vi "AlliGator GUI Actions.vi"(0 "AlliGator Q Elements in":T6[](array[typedef]), 1 "VI in":refnum<vi>, 2 "Script":bool, 5 "AlliGator IV DVR":refnum<data-value>, 7 "AlliGator Q Event in":T7=enum."GUI:Idle", 9 "Data":variant, 11 "error in (no error)":errorcluster, 12 "AlliGator Ctrl Refnums":T8) -> (3 "Script?":bool, 4 "AlliGator Q Elements out":T6[](array[typedef]), 6 "AlliGator IV DVR":refnum<data-value>, 10 "[Notebook Message]":T1[](array[typedef]) {"Message Style"."Font Size" min=6.0 step=1.0}, 14 "Quit?":bool, 15 "error out":errorcluster)   [LabVIEW 2021, in "AlliGator Action Engine.lvlib"]
doc: "Processes AlliGator GUI-related actions."
uses:
  AlliGator Action Engine.lvlib
  Internal Variables/AlliGator Internal Variables v2.ctl
  <vilib>/vision/Image Controls.llb/IMAQ Image.ctl
  Internal Variables/AlliGator Gate Image Set.ctl
  Files/AlliGator FLI Dataset Type.ctl
  Files/AlliGator Data Series Type.ctl
  Dual-Channel Datasets/AlliGator Dataset Channel.ctl
  Settings/AlliGator Gate Arithmetic.ctl
  Source Image/AlliGator Displayed Image.ctl
  Image/Named ROI Description.ctl
  Phasor Graph/AlliGator Decay Metadata v3.ctl
  Decay Analysis/Decay Preprocessing/AlliGator Decay Background Subtraction Info.ctl
  Decay Analysis/Decay Preprocessing/AlliGator Baseline Subtraction Method.ctl
  Graphs/XY Graph/XY Graph Plot Shift Parameters.ctl
  Graphs/XY Graph/XY Graph Plot Shift Method.ctl
  Decay Analysis/Decay Preprocessing/AlliGator Decay Extrapolation Parameters.ctl
  Phasor/Calibration Phasor (m, phi).ctl
  Phasor/Phasor Reference Series.ctl
  Phasor/Phasor Calibration Map v2.ctl
  Phasor/Phasor (g, s).ctl
  Phasor Graph/AlliGator Raw Phasor Plot Data v5.ctl
  Phasor/Phasor Standard Deviation Options.ctl
  Phasor Plot/AlliGator Phasor Multi-Harmonic Data.ctl
  Phasor/Phasor Harmonic Data.ctl
  Decay Fit Parameter Map/AlliGator Decay Fit Options & Parameters v4.ctl
  Fits/IRF(X)PSED/Decay Fit Options v4.ctl
  Fits/Decay Convolution/Decay Model.ctl
  Fits/Residual Type.ctl
  Fits/IRF(X)PSED/Fit Weights Type v2.ctl
  Fits/Non-linear Fitting Method v2.ctl
  Fits/Fit Calculation Method.ctl
  Fits/Non-linear Fitting Algorithm.ctl
  Decay Analysis/Decay Fit/AlliGator Decay Fit Parameter Constraints 2.ctl
  Fits/IRF(X)PSED/Decay Fit Parameters In List.ctl
  Fits/IRF(X)PSED/MLE Baseline Offset Type.ctl
  Decay Analysis/Decay Preprocessing/AlliGator Decay Preprocessing Parameters.ctl
  Fits/IRF(X)PSED/Decay Fit Parameters & Derived Quantities List v2.ctl
  Fits/IRF(X)PSED/Decay Fit Result Constraint.ctl
  Decay Fit Parameter Map/AlliGator Parameter Maps Data.ctl
  AlliGator Q Event.ctl
  GUI/AlliGator Ctrl Refnums.ctl
  GUI/AlliGator Other Ctrl Refnums.ctl
  GUI/AlliGator State Indicator.ctl
  GUI/AlliGator Main Window Tabs.ctl
  GUI/AlliGator Phasor Plot Ctrl Refnums.ctl
  GUI/AlliGator Phasor Graph Ctrl Refnums.ctl
  Phasor/Phasor Calibration Type.ctl
  GUI/AlliGator Dataset Ctrl Refnums.ctl
  GUI/AlliGator Registered Events Ctrl Refnums.ctl
  GUI/AlliGator Image Histogram Control Refnums.ctl
  Histograms/Linear Histogram Options.ctl
  Histograms/Histogram Bin Option.ctl
  Histograms/Histogram Bin Position.ctl
  Decay Fit Parameter Map/AlliGator Decay Fit Map Control Refnums.ctl
  Parameter Map/AlliGator Parameter Map Control Refnums.ctl
  AlliGator Q Element.ctl
  Notebook/Notebook Message Object.ctl
  Rich Text Box/Text Formatting.ctl
  Rich Text Box/Text Colors.ctl
  Rich Text Box/Text Style.ctl
  Rich Text Box/Text Alignment.ctl
  Rich Text Box/Text Format List.ctl
  Globals, Variables, Constants/AlliGator Variables List.ctl
  Settings/AlliGator Settings List.ctl
  Alligator Elements Order in Action Stack.ctl
  GUI/AlliGator Open Wndow Event Data.ctl
  GUI/AlliGator Windows List.ctl
  GUI/Open VI Options.ctl
  GUI/Embedded Progress Bar Q Element.ctl
  AlliGator State Indicators List.ctl
  GUI/AlliGator Set State Indicator Data.ctl
  Test Suites/AlliGator Test Data.ctl
  Globals, Variables, Constants/AlliGator Globals.vi
  Globals, Variables, Constants/AlliGator Abort.vi
  Variant/Variant to Data/Variant to Boolean.vi
  Fits/Abort Fit Global.vi
  Variant/Variant to Data/Variant to U16.vi
  Variant/Variant to Data/Variant to String.vi
  Variant/Variant to Data/Variant to I32.vi
  Source Image/AlliGator Source Image.lvlib
  GUI/AlliGator GUI.lvlib
  Globals, Variables, Constants/AlliGator Globals, Variables & Constants.lvlib
  Variant/Variant to Data/Variant to Data.lvlib
  Internal Variables/AlliGator Internal Variables.lvlib
  GUI/GUI.lvlib
  ROIs/AlliGator ROIs.lvlib
  Strings/Strings.lvlib
  Settings/AlliGator Settings.lvlib
  Notebook/Notebook.lvlib
  Scripts/AlliGator Scripts.lvlib
  Python Plugins API/AlliGator Python Plugins.lvlib
  Fits/Fits.lvlib
  Utilities/Utilities.lvlib
  Sound/Sound.lvlib
  Formula/Formula.lvlib
  Test Suites/AlliGator Test Suite.lvlib
  Phasor/Phasor.lvlib
  Image/Image.lvlib
  Decay Analysis/Decay Preprocessing/AlliGator Decay Preprocessing.lvlib
  Graphs/XY Graph/XY Graph Add-Ons.lvlib
  Phasor Graph/AlliGator Phasor Graph.lvlib
  Files/AlliGator Files.lvlib
  Phasor Plot/AlliGator Phasor Plot.lvlib
  Decay Analysis/Decay Fit/AlliGator Decay Fit.lvlib
  Decay Fit Parameter Map/AlliGator Decay Fit Parameter Map.lvlib
  Rich Text Box/Rich Text Box.lvlib
  Dual-Channel Datasets/AlliGator Dual-Channel Datasets.lvlib
  Histograms/Histogram Window.lvlib
  Parameter Map/AlliGator Parameter Map.lvlib
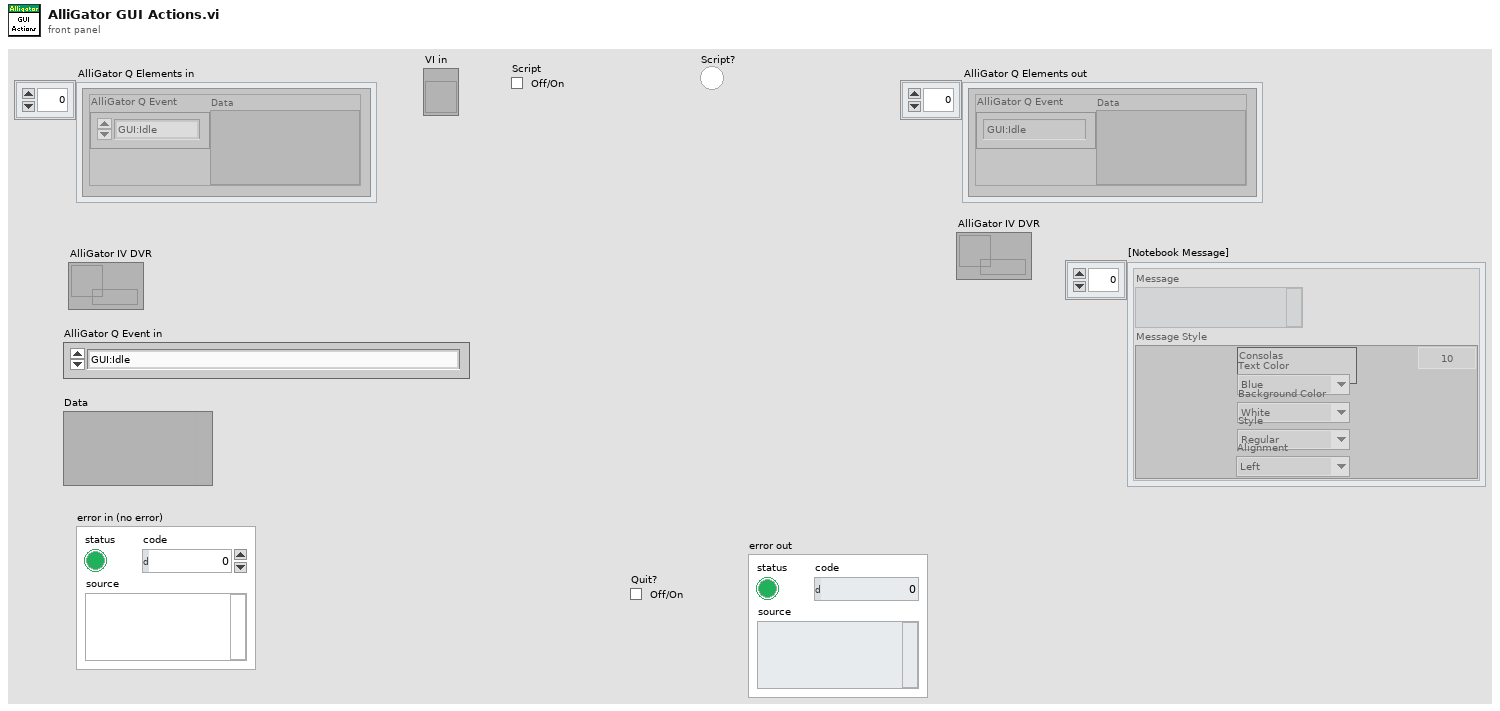
[diagram p1: front panel]
types:
  T1 = typedef "Notebook.lvlib/Notebook Message Object.ctl" = cluster{"Message":string, "Message Style":T2}
  T2 = typedef "Rich Text Box.lvlib/Text Formatting.ctl" = cluster{"Font":string, "Text Color":T3, "Background Color":T3, "Style":T4, "Font Size":dbl, "Alignment":T5}
  T3 = typedef "Rich Text Box.lvlib/Text Colors.ctl" = enum16{"Unchanged", "Black", "Blue", "Cyan", "Maroon", "Gray", "Violet", "Green", "Light Green", "Orange", "Yellow", "Magenta", "Red", "White"}
  T4 = typedef "Rich Text Box.lvlib/Text Style.ctl" = enum16{"Regular", "Bold", "Italic", "Underline", "Strikeout"}
  T5 = typedef "Rich Text Box.lvlib/Text Alignment.ctl" = enum16{"Left", "Right", "Center"}
  T6 = typedef "AlliGator Action Engine.lvlib/AlliGator Q Element.ctl" = cluster{"AlliGator Q Event":T7, "Data":variant}
  T7 = typedef "AlliGator Action Engine.lvlib/AlliGator Q Event.ctl" = enum16{"---- Files ----", "Files:Set Batch Export Files To Save", "Files:Set Dataset Loading & Pre-processing Options", "Files:Check #Frames in Dataset", "Files:Increment Frame Index", "Files:Open Mask Image", "Files:Open White Light Image", "Files:Open Single Dataset", "Files:New Folder of Folders Selected", "Files:Load File (all Types)_Scriptable", "Files:Move Flattened Series to Folders Series", "Files:Select Folder", "Files:Load FLI Dataset", "Files:Load Swiss SPAD 1 Dataset", "Files:Load Swiss SPAD 2 Dataset", "Files:Load .sdt FLI Dataset", "Files:Load .ptu FLI Dataset", "Files:Load .bin FLI Dataset", "Files:Load Single Gate Image Folder", "Files:Load I/m/phi Dataset (deprecated)", "Files:Load Single Image", "Files:Subtract Background File", "Files:Export FLI Dataset", "Files:Load HDF5 FLI Dataset", "Files:Set Destination File Path", "Files:Save Mask Image", "Files:Batch Conversion", "Files:New Folder Selected", "Files:Close FLI Dataset", "Files:Close FLI Dataset Series", "Files:Close White Light Image", "Files:Close Mask Image", "---- FLI Dataset ----", "FLI Dataset:Channel Arithmetic", "FLI Dataset:Export Average Lifetime Map as ASCII", "FLI Dataset:Export User-Defined Quantity Map as ASCII", "FLI Dataset:Python Function FLI Dataset Event", "FLI Dataset:ROI Analysis", "FLI Dataset:Tilted Logistic Square Gated IRF Characteristics Map", "FLI Dataset:Logistic Square Gated IRF Characteristics Map", "FLI Dataset:Square Gated IRF Characteristics Map", "FLI Dataset:Multi-ROI Single-Pixel Phasor Analysis", "FLI Dataset:Multi-ROI Single-Pixel NLSF Analysis", "FLI Dataset:All ROIs IRF Extraction", "FLI Dataset:All ROIs Decay Fit Non-Interactive (Fast + Individual IRF)", "FLI Dataset:All ROIs Phasor Analysis", "FLI Dataset:All ROIs Decay Fit", "FLI Dataset:Fluorescence Decay Statistics", "FLI Dataset:Update Decay Statistics Graph", "FLI Dataset:Get Decay from ROI", "FLI Dataset:All ROIs Average Lifetimes", "FLI Dataset:Save/Load Local IRFs", "FLI Dataset:Clear Local IRFs", "FLI Dataset:Phasor Calibration Maps (# Gates Series) Script", "FLI Dataset:Calibrated Phasor Map Series", "---- FLI Dataset Series ----", "FLI Dataset Series:Sum All Datasets in Series", "FLI Dataset Series:Add Dataset to Accumulated Dataset", "FLI Dataset Series:Display Accumulated Dataset", "FLI Dataset Series:Clear Dataset Series Sum", "FLI Dataset Series:Time-Series Analysis (NLSF)", "FLI Dataset Series:Time-Series Analysis (Phasor)", "---- Image ----", "Image:Update Image Profile Plots", "Image:Image Histogram Cursor Move", "Image:Image Histogram", "Image:Image Contrast", "Image:Set Image Histogram Cursor Move Flag", "Image:Clear Image Overlay", "Image:Use ROI as Search Area", "Image:Set ROI Diameter", "Image:Save Image Data as TIFF", "Image:Save Displayed Image with Overlay", "Image:Save Image Overlay Only", "Image:Save Image as Hot Pixel Mask", "Image:Change Source Image Color Palette", "Image:Copy Image to Clipboard", "Image:Source Image ROI Selection", "Image:Delete All ROIs", "Image:Delete All Unselected ROIs", "Image:Delete ROI", "Image:Merge All ROIs", "Image:Store ROI", "Image:Source Image ROI Storage", "Image:Export ROI Description to Notebook", "Image:Save ROI", "Image:Load ROI", "Image:Paste ROI Definition", "Image:Clear ROI", "Image:Identify ROIs in Mask Image", "Image:Create Complementary ROI", "Image:Create Contour ROI", "Image:Create ROI(s) from Pixels with Peak above Min_Scriptable", "Image:Create ROI(s) from Pixels with Intensity above Min_Scriptable", "Image:Compute ROI Statistics", "Image:Delete ROI(s) based on ROI Characteristics", "Image:Create ROI Grid", "Image:ROI to Individual Pixel ROIs", "Image:Python Function Source Image Event", "Image:Show Phasor Calibration Map ROI Centers", "Image:Convert ROI to Mask Image", "Image:Mouse Move", "Image:Mouse Up", "Image:Set Source Image Mouse Move Flag", "Image:Add Scale Bar Overlay", "Image:Delete Existing ROIs Option", "Image:Overlay ROI Median", "Image:Check Current ROI", "Image:Update True Pixel Value", "---- Decay ----", "Decay:Clear IRF/Reference Plot", "Decay:Add Decay to Graph", "Decay:Smoothen Plot", "Decay:Smoothen Plot Tail", "Decay:Average Selected Plots", "Decay:Extract IRF", "Decay:Optimal IRF Extraction", "Decay:Threshold IRF", "Decay:Fit to Model IRF", "Decay:Fit IRF to Square Gate", "Decay:Fit IRF to Logistic Square Gate", "Decay:Fit IRF to Tilted Logistic Square Gate", "Decay:Create Bounding Cursors Set", "Decay:Export Bounding Cursors Definition to Notebook", "Decay:Denoise Plot", "Decay:Compute Cumulative Function", "Decay:Use as Reference Decay", "Decay:Show Reference Decay/IRF", "Decay:Extrapolate Decay", "Decay:Create Head & Tail Bounding Cursors", "Decay:Store Cursor-defined Head & Tail Fractions", "Decay:Rebin Plot", "Decay:1-Normalize Decay", "Decay:[0-1]-Normalize Plot", "Decay:Straighten Decay", "Decay:Shift Decay", "Decay:Fold Decay", "Decay:Fit Decay", "Decay:Global Fit of Selected Decays", "Decay:Post Global Fit Script", "Decay:Add Global Fit Parameters to Graph", "Decay:Add Decay Parameter(s) to Plot (Graph)", "Decay:Export Decay to Phasor Graph", "Decay:Compute Average Lifetime", "Decay:Plot Convolution", "Decay:Graph Tip Strip Update", "---- Decay Statistics ----", "Decay Statistics:Tip Strip Update", "---- Intensity Time Trace ----", "Intensity Time Trace:Use File Timestamp", "Intensity Time Trace:Load Intensity Corrections File", "Intensity Time Trace:Clear Intensity Corrections File", "Intensity Time Trace:Tip Strip Update", "---- Phasor Plot ----", "Phasor Plot:Build Phasor Plot", "Phasor Plot:Change Phasor Plot Color Palette", "Phasor Plot:Adjust Phasor Plot Display Range", "Phasor Plot:Highlight Image ROI in Phasor Plot", "Phasor Plot:Save Phasor Plot Image with Overlay", "Phasor Plot:Export Complex Phasor Map", "Phasor Plot:Export Phasor Ratio Map", "Phasor Plot:Export Average Lifetime Map", "Phasor Plot:Compute Phase Lifetime Histogram", "Phasor Plot:Compute Phasor Ratio Histogram", "Phasor Plot:Compute Phase Lifetime vs Intensity Scatter Plot", "Phasor Plot:Weber 2-Component Decomposition", "Phasor Plot:Update Phasor Color Map Vertices", "Phasor Plot:Clear Phasor Overlay", "Phasor Plot:Use Segment Extremities as References", "Phasor Plot:Use UC/Segment Intersections as References", "Phasor Plot:Use UC/Principal Axis Intersections as References", "Phasor Plot:Use UC/Linear Fit Intersections as References", "Phasor Plot:Update Phasor Plot Reference", "Phasor Plot:Show Local Phasor Info in Phasor Plot", "Phasor Plot:Update Phasor Plot State", "Phasor Plot:Phasor Plot ROI Storage", "Phasor Plot:Phasor Plot ROI Selection", "Phasor Plot:Python Function Phasor Plot Event", "Phasor Plot:Overlay Phasor ROI, Ratio or Map in Source Image", "Phasor Plot:Compute Decay of Selected Phasors", "Phasor Plot:Phasor at Image Pixel", "Phasor Plot:Mouse Move", "Phasor Plot:Mouse Up", "Phasor Plot:Display Range Mouse Move", "Phasor Plot:Set Mouse Move Flag", "Phasor Plot:Update True Phasor Plot Value", "---- Phasor Graph ----", "Phasor Graph:Get Phasor Value", "Phasor Graph:Create New Phasor Plot Dialog", "Phasor Graph:Update Last Phasor Value", "Phasor Graph:Update Phasor (m, phi)", "Phasor Graph:Remove Single Phasor from Plot", "Phasor Graph:Add Single Phasor to Plot", "Phasor Graph:Remove Phasor Plot", "Phasor Graph:Remove Selected Phasor Plots", "Phasor Graph:Clear Phasor Data", "Phasor Graph:Clear Phasor Graph", "Phasor Graph:Cursor Move", "Phasor Graph:Draw Cursor Connecting Line", "Phasor Graph:Clear Cursor Connecting Line", "Phasor Graph:Find UC Intersection", "Phasor Graph:Use UC/Cursor-Defined Line Intersections", "Phasor Graph:Use Selected Plots Fitted Line/UC Intersections", "Phasor Graph:Use Selected Plots Principal Axis/UC Intersections", "Phasor Graph:Show Single Phasor", "Phasor Graph:Save Single Phasor Plot", "Phasor Graph:Save All Phasor Plots", "Phasor Graph:Load Phasor Plot(s)", "Phasor Graph:Phasor Multiplication", "Phasor Graph:Compute Average Phasor", "Phasor Graph:Compute Multiple Average Phasors (Selected Plots)", "Phasor Graph:Export Single Phasor Plot Phase Lifetimes", "Phasor Graph:Parameter 2 vs Parameter 1 Scatter Plot", "Phasor Graph:Use Cursor n Location", "Phasor Graph:Set Reference n to Current Phase Lifetime Value", "Phasor Graph:Set Reference n to Lifetime Value", "Phasor Graph:Set Cursor n Location", "Phasor Graph:Save Phasor Graph Image", "Phasor Graph:Update SEPL Plot", "Phasor Graph:Export Single Phasor Plot Data", "Phasor Graph:Export Selected Phasor Plots Data", "Phasor Graph:Python Function Phasor Graph Event", "Phasor Graph:Tip Strip Update", "---- Calibration ----", "Calibration:Set Calibration Type", "Calibration:Load/Save Phasor Calibration", "Calibration:Load/Save Phasor Calibration Series", "Calibration:Load/Save Phasor Calibration Map", "Calibration:Use as Calibration", "Calibration:Compute Optimal Calibration from Phasor References", "Calibration:Clear Phasor Calibration", "Calibration:Single Phasor Calibration Information", "Calibration:Use as Calibration Series", "Calibration:Use as Calibration Map", "Calibration:Clear Calibration Series", "Calibration:Phasor Calibration Series Information", "Calibration:Clear Calibration Map", "Calibration:Phasor Calibration Map Information", "Calibration:Apply Phasor Calibration", "Calibration:Update Single Plot Calibration", "Calibration:Update Multiple Plots Calibration", "Calibration:Clear Single Plot Calibration", "Calibration:Clear All Plots Calibrations", "Calibration:Clear Plot(s) Calibration(s)?", "---- Phasor Ratio ----", "Phasor Ratio:Clear Reference n", "Phasor Ratio:Toggle Selected Plot(s)  Lock to Reference 1", "Phasor Ratio:Use as Reference n", "Phasor Ratio:Send Reference n to Notebook", "Phasor Ratio:Toggle Selected Plot(s)  Lock to Reference 2", "Phasor Ratio:Compute Phasor Ratio at Mouse Location", "Phasor Ratio:Compute Phasor Plot's Average Phasor Ratio", "Phasor Ratio:Compute Time-Series Phasor Ratios", "Phasor Ratio:Fit Line to Phasor Ratio Plot", "Phasor Ratio:Save References", "Phasor Ratio:Load References", "Phasor Ratio:Update Phasor Reference 1", "Phasor Ratio:Update Phasor Reference 2", "Phasor Ratio:Move Cursor n to Reference n", "Phasor Ratio:Use as Phasor Reference 1 Lifetime", "Phasor Ratio:Use as Phasor Reference 2 Lifetime", "Phasor Ratio:Export Phasor Ratio Map as ASCII", "Phasor Ratio:Tip Strip Update", "---- Lifetime & Other Parameters Graph ----", "Lifetime:Compute Sliced Mean, SDV and CV Plots", "Lifetime:Plot Decay Shifts", "Lifetime:Plot Histogram", "---- Decay Fit Parameter Map ----", "Decay Fit Parameter Map:Export ROI NLSF Data as ASCII", "Decay Fit Parameter Map:Set Decay Fit Parameter Map Selection", "Decay Fit Parameter Map:Build Decay Fit Parameter Map", "Decay Fit Parameter Map:Change Decay Fit Parameter Map Color Palette", "Decay Fit Parameter Map:Export Decay Fit Parameter Map Data as ASCII", "Decay Fit Parameter Map:Export All Decay Fit Parameter Maps Data as ASCII", "Decay Fit Parameter Map:Selected Parameter Scatterplot", "Decay Fit Parameter Map:Parameter 2 vs Parameter 1 Scatterplot", "Decay Fit Parameter Map:Save Decay Fit Parameter Map Image", "Decay Fit Parameter Map:Save-Load IRFs & Fit Data", "Decay Fit Parameter Map:Update Local Decay Plots", "Decay Fit Parameter Map:Python Function Decay Fit Parameters Map Event", "Decay Fit Parameter Map:Overlay Decay Fit Parameter Map in Source Image", "Decay Fit Parameter Map:Selected Parameter vs Intensity Scatterplot", "Decay Fit Parameter Map:Mouse Up", "Decay Fit Parameter Map:Mouse Move", "Decay Fit Parameter Map:Display Range Mouse Move", "Decay Fit Parameter Map:Change Map Resolution", "Decay Fit Parameter Map:Variance Significance Maps", "Decay Fit Parameter Map:Fit Result Constraints Window", "---- Parameter Map ----", "Parameter Map:Export ROI Parameters Data as ASCII", "Parameter Map:Add Parameter Map Set", "Parameter Map:Delete Parameter Map Set", "Parameter Map:Update Parameter List", "Parameter Map:Build Parameter Map", "Parameter Map:Change Parameter Map Color Palette", "Parameter Map:Export Parameter Map Data as ASCII", "Parameter Map:Export All Parameter Maps Data as ASCII", "Parameter Map:Selected Parameter Scatterplot", "Parameter Map:Parameter 2 vs Parameter 1 Scatterplot", "Parameter Map:Selected Parameter vs Intensity Scatterplot", "Parameter Map:Save Parameter Map Image", "Parameter Map:Save-Load IRFs & Parameter Maps (TODO)", "Parameter Map:Set Parameter Map Selection", "Parameter Map:Python Function Parameter Map Event", "Parameter Map:Overlay Parameter Map in Source Image", "Parameter Map:Update Local Decay Plots", "Parameter Map:Mouse Up", "Parameter Map:Mouse Move", "Parameter Map:Display Range Mouse Move", "---- Generic Graph ----", "Generic Graph:Generic XY Graph Event", "Generic Graph:Python Function XY Graph Event", "Generic Graph:New Plot", "Generic Graph:Save Plot", "Generic Graph:XY Plot Histogram", "Generic Graph:Set XY Graph Plot Name", "Generic Graph:Set Last Cursor Style", "Generic Graph:Tip Strip Update", "---- GUI ----", "GUI:Start Script", "GUI:Type of Displayed Image Changed", "GUI:Gate Image Slide Changed", "GUI:Show Busy Icon", "GUI:Show Busy Icon & Abort Button", "GUI:Hide Busy Icon", "GUI:Hide Busy Icon & Abort Button", "GUI:Abort", "GUI:End Script", "GUI:Start Timing", "GUI:End Timing", "GUI:Set State Indicator", "GUI:Send Parameters JSON Strings to Clipboard", "GUI:Set Gate Step", "GUI:Idle", "GUI:Initialization", "GUI:Quit", "GUI:Increment Dataset Index", "GUI:Set Dataset Index to -1", "GUI:Time Series Slider Moved", "GUI:Time Series Slider Changed", "GUI:Toggle Playback or Loop", "GUI:Playback Script", "GUI:Set Phasor Frequency", "GUI:Open Window", "GUI:Start Test Script", "GUI:End Test Script", "GUI:Set Verbose Mode", "GUI:Set Verbose Settings Mode", "DEBUG"}
  T8 = typedef "AlliGator GUI.lvlib/AlliGator Ctrl Refnums.ctl" = cluster{"Other AlliGator Ctrl Refnums":T9, "Phasor Plot Ctrl Refnums":T10, "Phasor Graph Ctrl Refnums":T11, "Dataset Control Refnums":T12, "Registered Events Ctrl Refnums":T13, "Image Histogram Ctrl Refnums":T14, "Decay Fit Map Ctrl Refnums":T15, "Parameter Map Ctrl Refnums":T16}
  T9 = typedef "AlliGator GUI.lvlib/AlliGator Other Ctrl Refnums.ctl" = cluster{"State Indicators":refnum<vi>, " Progress Bar":refnum<vi>, "Decay Graph Active":refnum<vi>, "Decay Statistics Bin":refnum<vi>, "Time Step":refnum<vi>, "Use File Timestamp":refnum<vi>, "Tab Control":refnum<vi>, "CPU":refnum<vi>, "Abort Fit":refnum<vi>, "Dataset File/Folder Path":refnum<vi>, "Abort ROI Creation":refnum<vi>, "Event LED":refnum<vi>, "Dataset File/Folder Path 2":refnum<vi>, "Dataset File/Folder Path 3":refnum<vi>, "Dataset File/Folder Path 4":refnum<vi>, "Dataset File/Folder Path 5":refnum<vi>, "Dataset File/Folder Path 6":refnum<vi>, "Dataset File/Folder Path 7":refnum<vi>, "Dataset File/Folder Path 8":refnum<vi>, "Dataset File/Folder Path 9":refnum<vi>, "Dataset File/Folder Path 10":refnum<vi>, "Dataset File/Folder Path 11":refnum<vi>}
  T10 = typedef "AlliGator GUI.lvlib/AlliGator Phasor Plot Ctrl Refnums.ctl" = cluster{"Phasor Ratio":refnum<vi>, "Modulus Lifetime":refnum<vi>, "Phasor at cursor (m, phi)":refnum<vi>, "Phase Lifetime":refnum<vi>, "Phasor at cursor (g, s)":refnum<vi>, "Phasor Plor Average Lifetime":refnum<vi>, "Phasor Plot Active":refnum<vi>, "Save Phasor Plot":refnum<vi>, "Image Overlay Color":refnum<vi>, "Phasor Plot Color Scale":refnum<vi>, "Reference 1 Button":refnum<vi>, "Reference 2 Button":refnum<vi>, "True Phasor Plot Value":refnum<vi>}
  T11 = typedef "AlliGator GUI.lvlib/AlliGator Phasor Graph Ctrl Refnums.ctl" = cluster{"Phasor Ratio":refnum<vi>, "Modulus Lifetime":refnum<vi>, "Phasor at cursor (m, phi)":refnum<vi>, "Phase Lifetime":refnum<vi>, "Phasor at cursor (g, s)":refnum<vi>, "Phasor Graph Average Lifetime":refnum<vi>, "Phasor Graph Active":refnum<vi>, "Save Phasor Graph":refnum<vi>, "Phasor Frame Slide":refnum<vi>, "Single Step Phasor":refnum<vi>, "Calibration Type":refnum<vi>, "Show Line":refnum<vi>, "Phase Lifetime 1":refnum<vi>, "Phase Lifetime 2":refnum<vi>, "Phasor Graph Frequency":refnum<vi>, "Phasor Reference 1 Control":refnum<vi>, "Phasor Reference 2 Control":refnum<vi>, "Calibration Lifetime":refnum<vi>, "Phase Lifetime SDV":refnum<vi>, "Average Lifetime SDV":refnum<vi>, "Phasor Ratio SDV":refnum<vi>, "Modulus Lifetime SDV":refnum<vi>}
  T12 = typedef "AlliGator GUI.lvlib/AlliGator Dataset Ctrl Refnums.ctl" = cluster{"Current Data":refnum<vi>, "Gate Image Slide":refnum<vi>, "Time Point Slide":refnum<vi>, "Current Time Stamp":refnum<vi>, "Save Image":refnum<vi>, "Displayed Image":refnum<vi>, "Overlay Mode":refnum<vi>, "Phasor Overlay Color":refnum<vi>, "Image Color Scale":refnum<vi>, "Use ROI as Search Area":refnum<vi>, "Source Image ROI Color":refnum<vi>, "True Pixel Value":refnum<vi>}
  T13 = typedef "AlliGator GUI.lvlib/AlliGator Registered Events Ctrl Refnums.ctl" = cluster{"Time Point Slider":refnum<vi>, "Phasor Plot Display Range":refnum<vi>, "Decay Graph":refnum<vi>, "Decay Statistics Graph":refnum<vi>, "Intensity Time Trace":refnum<vi>, "Phasor Graph":refnum<vi>, "Phasor Ratio Graph":refnum<vi>, "Lifetime Graph":refnum<vi>, "Phasor Plot Display":refnum<vi>, "Source Image Display":refnum<vi>, "Decay Fit Parameter Map Display Range":refnum<vi>, "Decay Fit Parameter Map Display":refnum<vi>, "Parameter Map Display Range":refnum<vi>, "Parameter Map Display":refnum<vi>, "Phasor Plot Display Range":refnum<vi>}
  T14 = typedef "AlliGator GUI.lvlib/AlliGator Image Histogram Control Refnums.ctl" = cluster{"Image Histogram":refnum<vi>, "Image Histogram Options":refnum<vi>, "Image Histogram Active":refnum<vi>, "Image Histogram Upper Percentile":refnum<vi>, "Image Histogram Lower Percentile":refnum<vi>, "Auto-Adjust Contrast":refnum<vi>}
  T15 = typedef "AlliGator Decay Fit Parameter Map.lvlib/AlliGator Decay Fit Map Control Refnums.ctl" = cluster{"Decay Fit Parameter Map Color Scale":refnum<vi>, "Decay Fit Parameter":refnum<vi>, "Max Parameter":refnum<vi>, "Min Parameter":refnum<vi>, "Decay Fit Parameter Map Display":refnum<vi>, "Decay Fit Parameter Map Display Range":refnum<vi>, "Decay Parameter Map X":refnum<vi>, "Decay Parameter Map Y":refnum<vi>, "Decay Parameter Map Value":refnum<vi>}
  T16 = typedef "AlliGator Parameter Map.lvlib/AlliGator Parameter Map Control Refnums.ctl" = cluster{"Parameter Map Color Scale":refnum<vi>, "Map Parameter":refnum<vi>, "Max Parameter":refnum<vi>, "Min Parameter":refnum<vi>, "Parameter Map Display":refnum<vi>, "Parameter Map Display Range":refnum<vi>, "Parameter Map Set":refnum<vi>, "Parameter Map X":refnum<vi>, "Parameter Map Y":refnum<vi>, "Parameter Map Value":refnum<vi>}
  T17 = typedef "Notebook.lvlib/Text Format List.ctl" = enum16{"Message", "Result", "Error", "Setting", "Verbose", "Warning"}
  T18 = typedef "AlliGator Globals, Variables & Constants.lvlib/AlliGator Variables List.ctl" = enum16{"---- GUI ----", "GUI:Initialization Status", "GUI:State Indicators Refnum", "GUI:Original AlliGator Menu Items", "GUI:Current Action Loop State", "GUI:Script in progress", "GUI:Playback", "GUI:Loop Playback", "GUI:Search ROI Used", "GUI:Search ROI", "Decay Graph Max Legend Size", "Intensity Graph Max Legend Size", "Decay Statistics Graph Max Legend Size", "Phasor Graph Max Legend Size", "Phasor Ratio Graph Max Legend Size", "Lifetime Graph Max Legend Size", "---- Files ----", "Files:Export Dataset Frames as Individual Files", "Files:Show Batch Export Help Balloons", "Files:Frames in Dataset", "Files:ptu File Frame Start Indices", "Files:Current Frame in Dataset", "Files:Current Frame Timestamp", "Files:Dataset Loaded", "Files:Dataset Metadata", "Files:Dataset Channel", "Files:Dataset Data Description", "Files:Background Dataset Metadata", "Files:Background Dataset Channel", "Files:Background Dataset Data Description", "Files:Background File Subtraction", "Files:Background File Path", "Files:Background File Pile-up Correction", "Files:Background File Pixel Well Capacity", "Files:Background File Scaling Factor", "Files:Current Dataset Load Settings", "Files:Dataset Path", "Files:ICCD-specific Information", "Files:Macrotime Gate Separation", "------ Python Plugins ------", "Python Plugins:Information", "Python Plugins:Python Session", "Python Plugins:Valid Python Session?", "---- Source Image ----", "Source Image:ROIs", "Source Image:Current ROI", "Source Image:ROI Event Refnum", "X_Source Image:Display Range", "X_Source Image:Palette Information", "X_Source Image:Type of Displayed Image", "X_Time Gate Slider", "Source Image:Palette List", "Source Image:Scale", "Source Image:ROI Overlay Color", "Source Image:Overlay to Erase", "Source Image:Is Displayed Image Accumulated", "Source Image:White Light Image Modified", "Source Image:Mask Image Modified", "---- Image Profile Window ----", "Image Profile:Window Event Refnum", "Image Profile:IntensityType", "Image Profile:Intensity Average Type", "Image Profile:Intensity-weighted SDV", "Image Profile:Box Profile Type", "Image Profile:Window Open", "Image Profile:Plotted Fit Parameter", "------ Phasor Graph -------", "Phasor Graph:Show Line", "---- Phasor Plot ---", "Phasor Plot:Parameters Changed", "Phasor Plot:FLI Dataset Modified since last Calculation", "Phasor Harmonics Data", "Selected Phasor Harmonics", "Phasor Harmonic Manager Event Refnum", "Phasor Plot:ROIs", "Phasor Plot:Current ROI", "Phasor Plot:ROI Event Refnum", "Phasor Plot:Image Reference Points", "Phasor Plot:Computed", "Phasor Plot:Palette Information", "Phasor Plot:Palette List", "Phasor Plot:Phasor Ratio Palette Information", "Phasor Plot:Phasor Ratio Palette List", "Phasor Plot:Image Scale", "Phasor Plot:Image Overlay to Erase", "Phasor Plot:Image Elements to Update", "Phasor Plot:Current Calculation Parameters", "Phasor Plot:Current Calibration Options", "Phasor Plot:Reset Cumulated Phasor Plot", "Phasor Plot:Reference 1", "Phasor Plot:Lifetime Reference 1", "Phasor Plot:Reference 1 Frequency", "Phasor Plot:Reference 2", "Phasor Plot:Lifetime Reference 2", "Phasor Plot:Reference 2 Frequency", "---- Decay Analysis ----", "Number of Selected Decays to Fit", "LS Fit Results", "LAR Fit Results", "BS Fit Results", "Last Decay Max - Min", "Best Fit Parameters", "Best Fit Parameter Names", "Actual Size X", "Actual Size Y", "Binning X", "Binning Y", "Actual # Gates", "Dataset Number", "Gates to...", "Gates Skipped", "Gates to keep", "Gate Step", "Gate Separation", "Reversed Gates", "Pile-up Correction", "Pixel Well Capacity", "Background Subtracted", "Background Subtraction Method", "Background Definition Range", "Background File (deprecated)", "Number of Dataset Accumulated", "Array of Accumulated Dataset Paths", "Do Averaged Datasets", "Destination File Path", "Process Plot Target", "Use 1/D as Phasor Frequency", "---- Decay Fit Parameter Map -----", "Decay Fit Parameter Map:Palette Information", "Decay Fit Parameter Map:Palette List", "Decay Fit Parameter Map:X Resolution", "Decay Fit Parameter Map:Y Resolution", "Decay Fit Parameter Map:Use Decay Fit Result Constraints", "Decay Fit Parameter Map:Decay Fit Result Constraints", "Decay Fit Parameter Map:Decay Fit Result Constraints Applied", "---- Parameter Map ----", "Parameter Map:Palette Information", "Parameter Map:Palette List", "------- Local Decay Window ---------", "Local Decay Graph Window:Event Refnum", "Local Decay Graph Window:Use normalized IRF for convolution", "----- Miscellaneous ----", "Misc:Skippable Dialog Windows Status"}
  T19 = typedef "AlliGator Settings.lvlib/AlliGator Settings List.ctl" = enum16{"GUI:Visible Settings Tab", "GUI:Last Run Version", "Source Image:Use Image Histogram for Contrast", "Source Image:Low Count Pixels Rejection Options", "Source Image:High Count Pixels Rejection Options", "Source Image:Use Image Brightness", "Source Image:Blend Overlay with Image Background", "Source Image:Use Fixed ROI Diameter", "Source Image:ROI Diameter", "Source Image:ROI Center Color", "Source Image:Peak Threshold", "Source Image:Intensity Threshold", "Source Image:Image Binning Options", "Source Image:Image Smoothing Options", "Source Image:Image Histogram Active", "Source Image:Invert Binary Mask", "Source Image:Hot Pixel Removal", "Source Image:Overlay Analyzed ROI Center", "Source Image:Auto-Adjust Contrast", "Source Image:Histogram Lower Percentile", "Source Image:Histogram Upper Percentile", "Source Image:Save Source Image", "Source Image:Scale Bar Options", "Source Image:Image Resolution (Pixel Size)", "Source Image:Flatfield Correction", "Source Image:Show Dead Left Columns Correction", "Source Image:Dead Left Columns Correction", "Source Image:Image Pre-Processing Operations Order", "Source Image:Overlay ROI Median", "Source Image:Median Overlay Color", "Data Information:Gate Width", "Data Information:Nanotime Gate Separation", "Data Information:Macrotime Gate Separation", "Data Information:Gate Step", "Data Information:# Gates", "Data Information:Gate Image Exposure", "Data Information:Gate Image Integration", "Data Information:Gates to Skip", "Data Information:Gates to Keep", "Data Information:Define Gates to", "Data Information:Channel Name", "Data Information:Available Channel Names", "Data Information:Channel Arithmetic", "Data Information:Background File Subtraction", "Data Information:Background File", "Data Information:Background Scaling Factor", "Data Information:Background Pile-up Correction", "Data Information:Background Pixel Well Capacity", "Data Information:Laser Period", "Data Information:SYNC Period", "Data Information:Pile-up Correction", "Data Information:Pixel Well Capacity", "Data Information:Dataset Scaling Factor", "Fluorescence Decay_Decay Pre-Processing:Reverse Gates", "Fluorescence Decay_Decay Pre-Processing:Verbose Decay Pre-Processing", "Fluorescence Decay_Decay Pre-Processing:Use Decay Pre-Processing", "Fluorescence Decay_Decay Pre-Processing:Background Subtraction", "Fluorescence Decay_Decay Pre-Processing:Background Definition Range", "Fluorescence Decay_Decay Pre-Processing:Baseline Subtraction Method", "Fluorescence Decay_Decay Pre-Processing:Decay Pre-Processing Operations Order", "Fluorescence Decay_Decay Pre-Processing:Smoothing Parameter", "Fluorescence Decay_Decay Pre-Processing:Shift Decay", "Fluorescence Decay_Decay Pre-Processing:Decay Shift Parameters", "Fluorescence Decay_Decay Pre-Processing:Fold Decay", "Fluorescence Decay_Decay Pre-Processing:# Folds", "Fluorescence Decay_Decay Pre-Processing:1-Normalize Decay", "Fluorescence Decay_Decay Pre-Processing:[0-1]-Normalize Decay", "Fluorescence Decay_Decay Pre-Processing:Smoothen Decay", "Fluorescence Decay_Decay Pre-Processing:Extrapolate Decay", "Fluorescence Decay_Decay Pre-Processing:Use Periodicity", "Fluorescence Decay_Decay Pre-Processing:Use Cursors", "Fluorescence Decay_Decay Pre-Processing:Tail Fraction", "Fluorescence Decay_Decay Pre-Processing:Head Fraction", "Fluorescence Decay_Decay Pre-Processing:Additional Points", "Fluorescence Decay_Decay Pre-Processing:Straighten Decay", "Fluorescence Decay_Decay Pre-Processing:Constant Background", "Fluorescence Decay_Decay Pre-Processing:Pixel-Normalize Decay", "Fluorescence Decay_Advanced Analysis:Extract IRF instead of Decay", "Fluorescence Decay_Advanced Analysis:IRF Extraction Options", "Fluorescence Decay_Advanced Analysis:IRF Optimization Options", "Fluorescence Decay_Advanced Analysis:Square Pulse Options", "Fluorescence Decay_Advanced Analysis:IRF Order", "Fluorescence Decay_Advanced Analysis:IRF Time Constants", "Fluorescence Decay_Advanced Analysis:Wavelet Analysis Options", "Fluorescence Decay_Advanced Analysis:Average Lifetime Options", "Fluorescence Decay_Fit Options:Fit Options", "Fluorescence Decay_Fit Options:Use Legacy Fitting Approach", "Fluorescence Decay_Fit Options:Use Data Information Laser Period", "Fluorescence Decay_Fit Parameters:Displayed Fit Parameters", "Fluorescence Decay_Fit Parameters:Fit Parameter Constraints", "Fluorescence Decay_Fit Parameters:Export Tabulated Results", "Fluorescence Decay_Fit Parameters:MLE Baseline Offset Type", "Fluorescence Decay_Fit Parameters:MLE Baseline Offset", "Fluorescence Decay_Fit Parameters:Guess Parameter Names", "Fluorescence Decay_Fit Parameters:Guess Parameter Values", "Fluorescence Decay_Fit Parameters:Guess Parameters Options", "Fluorescence Decay_Fit Parameters:Optimal Offset Selection Criterion", "Fluorescence Decay_Styles:Show Last Decay Only", "Fluorescence Decay_Styles:Decay Graph Color Array", "Fluorescence Decay:Decay Graph Active", "Fluorescence Decay Statistics:Min Peak Value", "Fluorescence Decay Statistics:Reject Low Decay Peak Pixels", "Fluorescence Decay Statistics:Reject High Decay Peak Pixels", "Fluorescence Decay Statistics:Max Peak Value", "Time Traces:Use File Timestamp", "Time Traces:Time Step", "Time Traces:Use Intensity Correction File", "Time Traces:Intensity Correction File", "Phasor Plot:Phasor Plot Smoothing Options", "Phasor Plot:Phasor Plot Size", "Phasor Plot:Phasor Plot Graphics Options", "Phasor Plot:Cumulative Phasor Plot", "Phasor Plot:Use Phasor Brightness", "Phasor Plot:Blend Overlay with Phasor Background", "Phasor Plot:Save Phasor Plot", "Phasor Plot:Show References", "Phasor Plot:Phasor Ratio Decay Range", "Phasor Plot:Exponential Fading", "Phasor Plot:Phasor Ratio Reference Colors", "Phasor Plot:Reference Radius", "Phasor Plot:Show Color Map Vertices", "Phasor Plot:Phasor Plot Active", "Phasor Plot:Phasor Ratio Color Map Type", "Phasor Plot:Phasor Ratio Color Map", "Phasor Plot:Phasor Ratio Display Range", "Phasor Plot:Selected Image ROI(s)", "Phasor Plot:All Image ROIs", "Phasor Plot:Selected Phasor Plot ROI(s)", "Phasor Plot:All Phasor Plot ROIs", "Phasor Plot:Phasor Ratio Color-Coded Quantity", "Phasor Plot:Store Phasor Harmonics", "Phasor Plot:Draw Reference Segment", "Phasor Plot:User-Defined Quantity", "Phasor Plot:Color Scale High Color", "Phasor Plot:Color Scale Low Color", "Phasor Plot:Intensity-weighted Phasor Plot", "Phasor Graph:Phasor Frequency", "Phasor Graph:Phasor Ratio Type", "Phasor Graph:Pixel-level Phasor Computation", "Phasor Graph:Save Phasor Graph", "Phasor Graph:Phasor Graph Active", "Phasor Graph:Phasor SDV Options", "Phasor Graph:Intensity-weighted Phasor Graph", "Phasor Graph:Define Shortest Lifetime as", "Phasor Calibration:Use Backup Calibration if needed", "Phasor Calibration:Backup Calibration Type", "Phasor Calibration:Calibration Type", "Phasor Calibration:Calibration Lifetime", "Phasor Calibration:Calibration Map Algorithm", "Single-Exponential Phasor Locus (SEPL):Gate Parameters", "Single-Exponential Phasor Locus (SEPL):User-defined Gate", "Single-Exponential Phasor Locus (SEPL):User-defined IRF", "Single-Exponential Phasor Locus (SEPL):Phasor Parameters", "Single-Exponential Phasor Locus (SEPL):Decay & IRF Parameters", "Single-Exponential Phasor Locus (SEPL):Display Parameters", "Lifetime Analysis:Decay Analysis Parameters", "Lifetime Analysis:Lifetime Map Active", "Plugins:Python Settings", "Miscellaneous:Verbose Mode", "Miscellaneous:Beep after Script", "Miscellaneous:Saved Image File Format", "Miscellaneous:Exported Gate Image Settings", "Miscellaneous:Include Loading in Timing", "Miscellaneous:Verbose Settings Mode", "Miscellaneous:Histogram Options", "Miscellaneous:Beep on Error", "Miscellaneous:# Logical Processors Used", "Miscellaneous:ROI Description Max Characters", "Miscellaneous:Verbose Error Mode", "Miscellaneous:Transparent Mask Color"}
  T20 = typedef "AlliGator Action Engine.lvlib/Alligator Elements Order in Action Stack.ctl" = enum16{"Enqueue 2 AFTER 1", "Enqueue 2 BEFORE 1"}
  T21 = typedef "AlliGator GUI.lvlib/AlliGator Open Wndow Event Data.ctl" = cluster{"AlliGator Windows":T22, "Open Window Options":T23}
  T22 = typedef "AlliGator GUI.lvlib/AlliGator Windows List.ctl" = enum16{"AlliGator Window", "Settings Window", "Notebook Window", "Dataset Information Window", "Source Image ROI Manager Window", "Phasor Plot ROI Manager Window", "Phasor Harmonic Manager Window", "Histogram Window", "Image Profile Window", "Local Decay Window", "About Window", "Batch Conversion Window", "Shot Noise Influence on Average Lifetime", "Fit Method Benchmark", "Camera Noise Influence on Lifetime", "AlliGator Alias Definition", "Fit Result Constraints Window"}
  T23 = typedef "GUI.lvlib/Open VI Options.ctl" = cluster{"Bring To Front (T)":bool, "Start Hidden? (F)":bool, "Activate? (T)":bool}
  T24 = typedef "GUI.lvlib/Embedded Progress Bar Q Element.ctl" = cluster{"Action":string, "Value":dbl}
  T25 = typedef "AlliGator Action Engine.lvlib/AlliGator State Indicators List.ctl" = enum16{"Phasor Calibration Defined", "Phasor Calibration Series Defined", "Phasor Calibration Map Defined", "Phasor Reference 1 Defined", "Phasor Reference 2 Defined", "Lifetime Reference 1 Defined", "Lifetime Reference 2 Defined", "Phasor Calibration Used", "Phasor Calibration Series Used", "Phasor Calibration Map Used", "Dataset Update Needed", "Phasor Plot Update Needed", "Reference/IRF Defined", "Individual IRFs Defined"}
  T26 = typedef "AlliGator GUI.lvlib/AlliGator Set State Indicator Data.ctl" = cluster{"State Indicators List":T25, "ON/OFF":bool, "# Defined IRFs":i32}
  T27 = typedef "AlliGator Source Image.lvlib/AlliGator Displayed Image.ctl" = enum16{"Single Gate", "Sum of All Gates", "Max of All Gates", "Min of All Gates", "-", "White Ligth Image", "Mask Image"}
  T28 = enum16{"Store Test Name", "Store Test Result", "Read Test Result"}
  T29 = typedef "AlliGator Test Suite.lvlib/AlliGator Test Data.ctl" = cluster{"Test String":string, "error":errorcluster, "Status":bool}
  T30 = typedef "AlliGator Files.lvlib/AlliGator Data Series Type.ctl" = enum16{"Not a Supported Series", "Gate Images Folder Series", "SwissSPAD 2 Dataset Series", "B&H FLI Dataset Series", "PicoQuant PTU FLI Dataset Series", "PicoQuant BIN FLI Dataset Series", "Piccolo hist BIN FLI Dataset Series", "HDF5 FLI Dataset Series"}
  T31 = typedef "AlliGator Displayed Image.ctl" = enum16{"Single Gate", "Sum of All Gates", "Max of All Gates", "Min of All Gates", "-", "White Ligth Image", "Mask Image"}
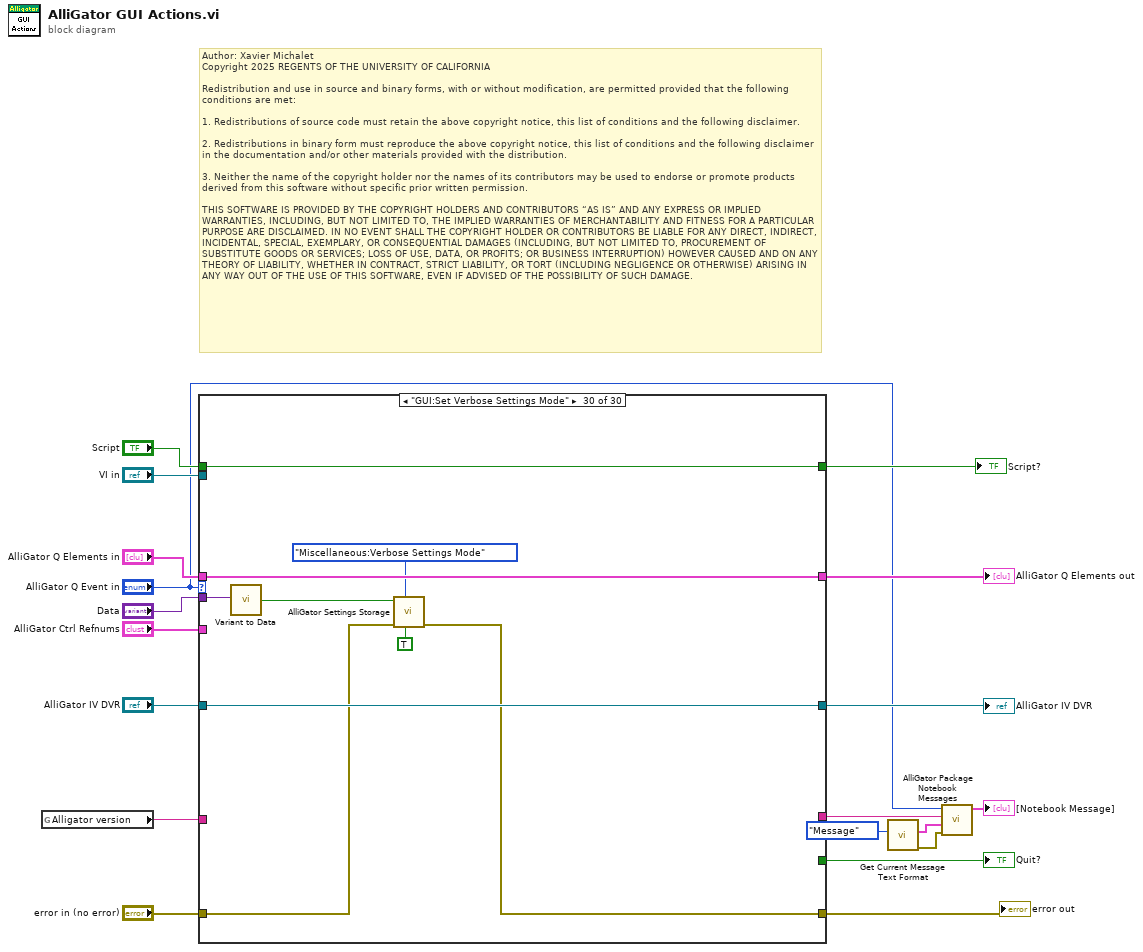
[diagram p0: block diagram]
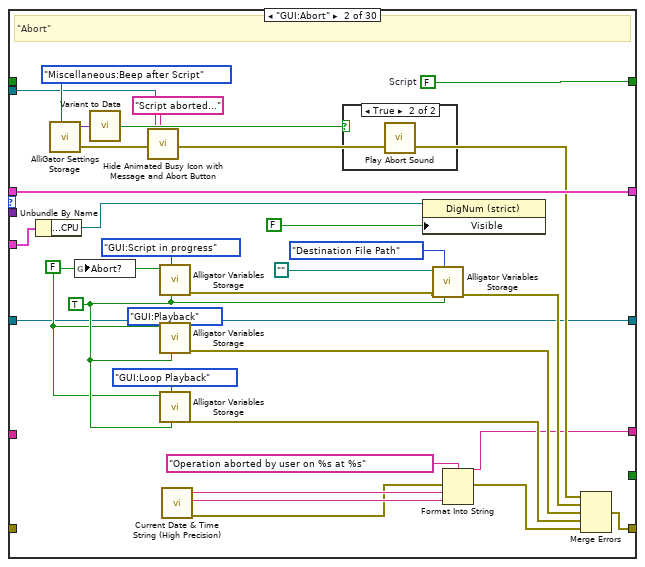
[diagram p3: hidden frame]
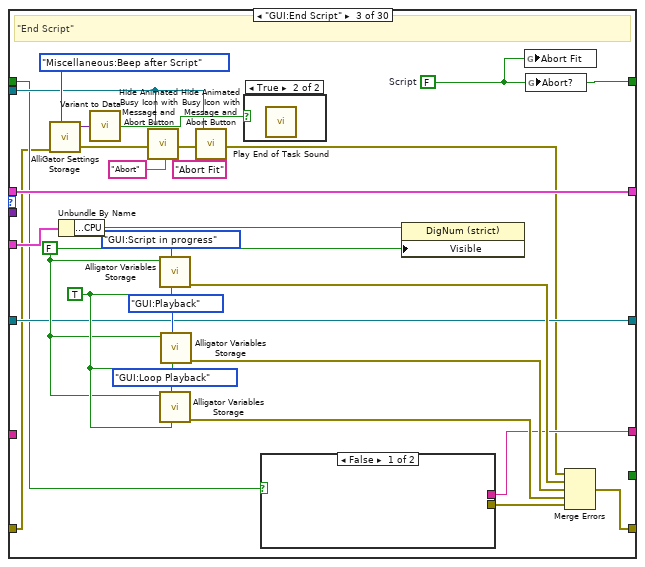
[diagram p5: hidden frame]
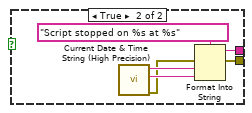
[diagram p6: hidden frame]
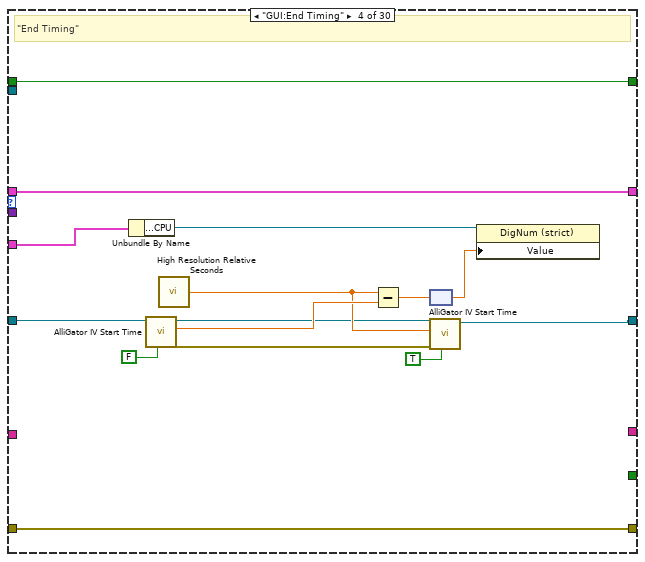
[diagram p8: hidden frame]
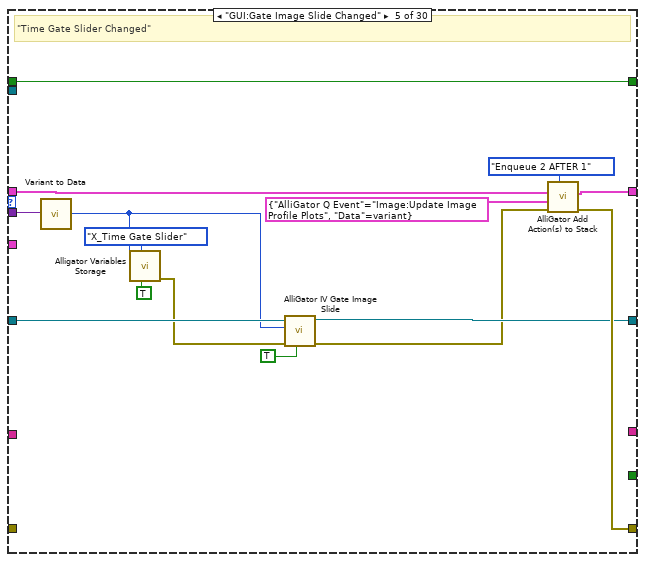
[diagram p9: hidden frame]
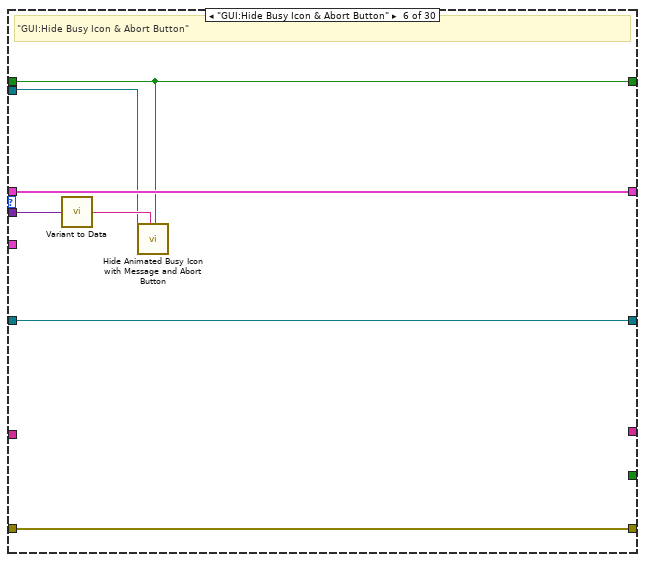
[diagram p10: hidden frame]
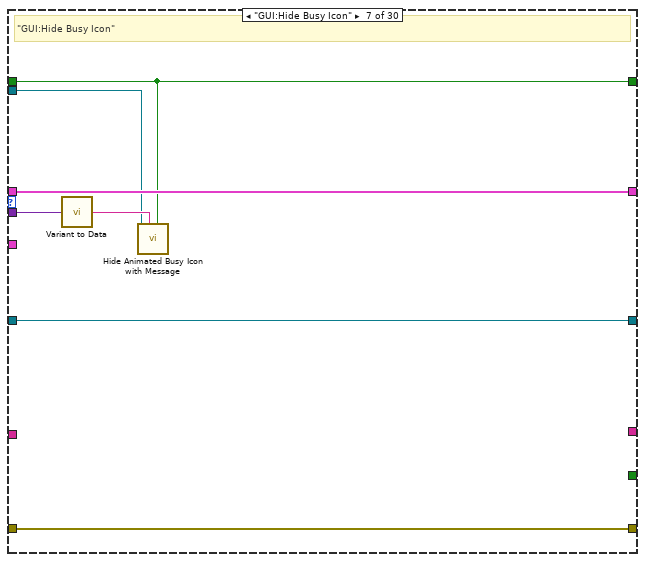
[diagram p11: hidden frame]
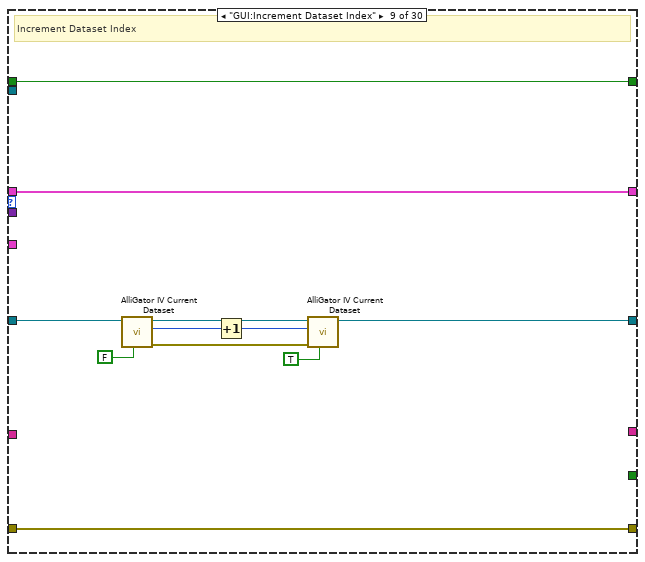
[diagram p13: hidden frame]
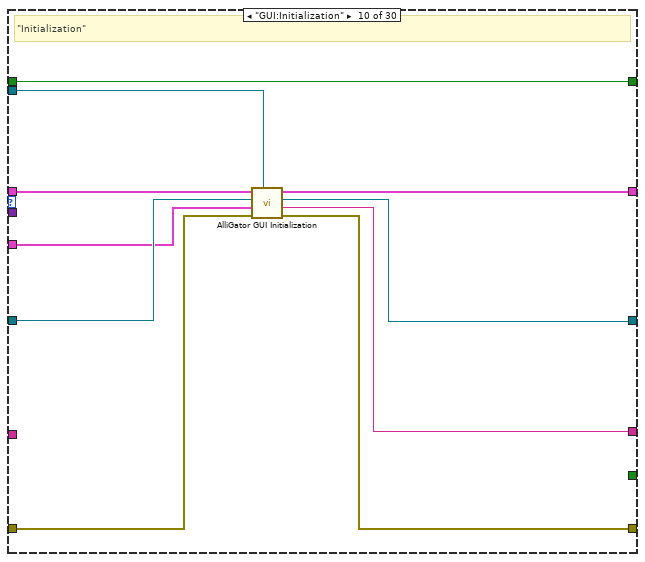
[diagram p14: hidden frame]
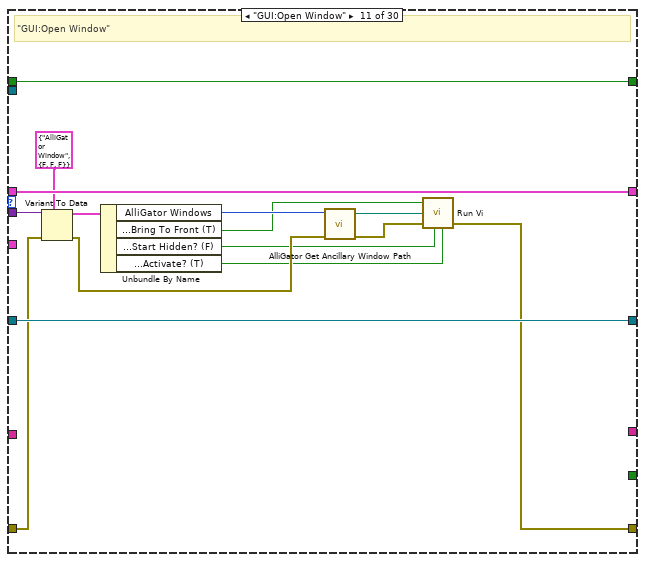
[diagram p15: hidden frame]
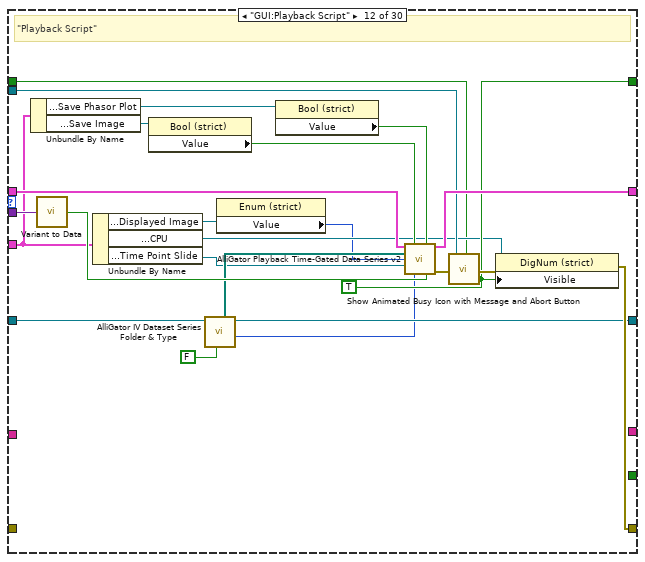
[diagram p16: hidden frame]
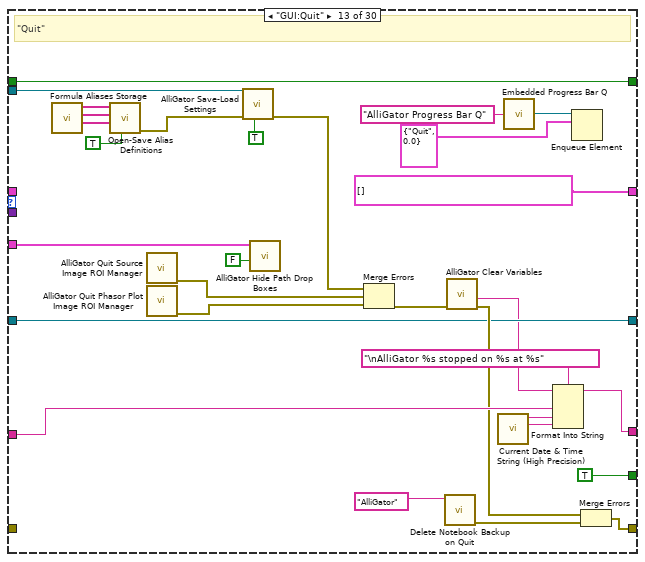
[diagram p17: hidden frame]
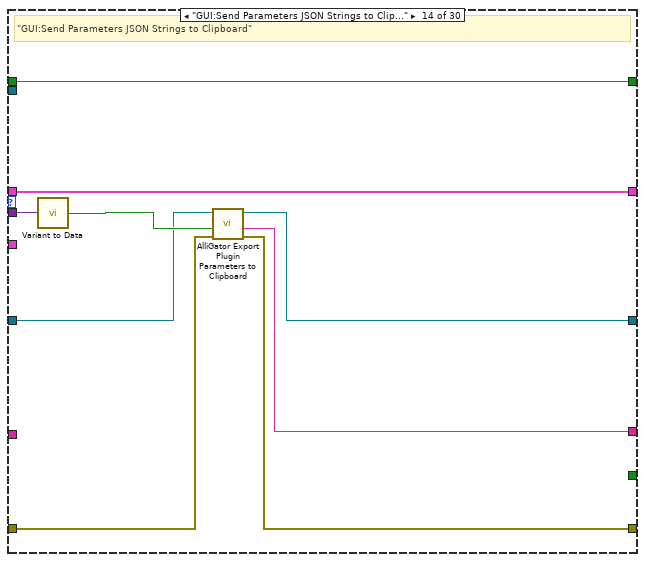
[diagram p18: hidden frame]
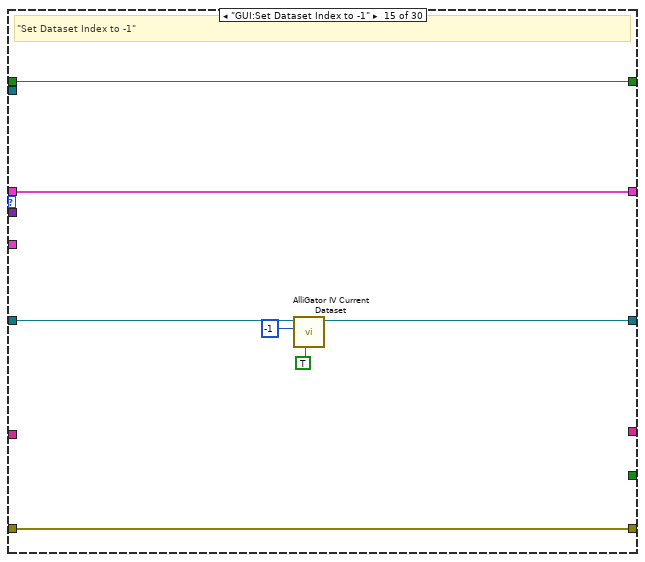
[diagram p19: hidden frame]
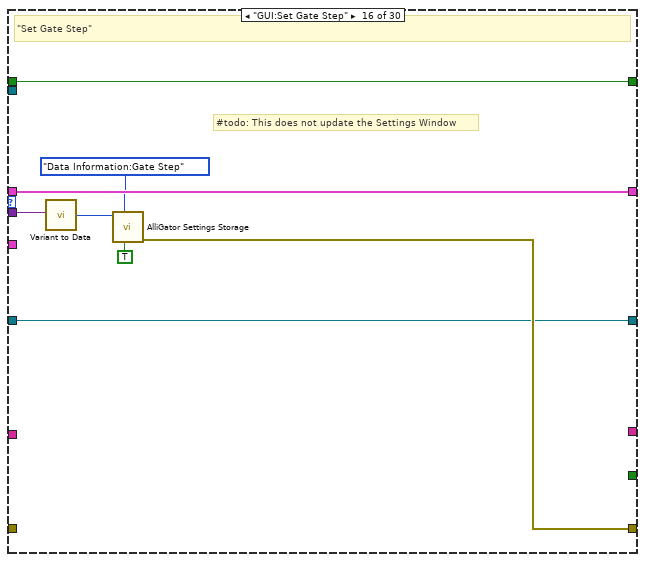
[diagram p20: hidden frame]
diagram:
  # "Author: Xavier Michalet\nCopyright 2025 REGENTS OF THE UNIVERSITY OF CALIFORNIA\n\nRedistribution and use in source and binary forms, with or without modification, are permitted provided that the following conditions are met:\n\n1. Redistributions of source code must retain the above copyright notice, this list of conditions and the following disclaimer.\n\n2. Redistributions in binary form must reproduce the above copyright notice, this list of conditions and the following disclaimer in the documentation and/or other materials provided with the distribution.\n\n3. Neither the name of the copyright holder nor the names of its contributors may be used to endorse or promote products derived from this software without specific prior written permission.\n\nTHIS SOFTWARE IS PROVIDED BY THE COPYRIGHT HOLDERS AND CONTRIBUTORS “AS IS” AND ANY EXPRESS OR IMPLIED WARRANTIES, INCLUDING, BUT NOT LIMITED TO, THE IMPLIED WARRANTIES OF MERCHANTABILITY AND FITNESS FOR A PARTICULAR PURPOSE ARE DISCLAIMED. IN NO EVENT SHALL THE COPYRIGHT HOLDER OR CONTRIBUTORS BE LIABLE FOR ANY DIRECT, INDIRECT, INCIDENTAL, SPECIAL, EXEMPLARY, OR CONSEQUENTIAL DAMAGES (INCLUDING, BUT NOT LIMITED TO, PROCUREMENT OF SUBSTITUTE GOODS OR SERVICES; LOSS OF USE, DATA, OR PROFITS; OR BUSINESS INTERRUPTION) HOWEVER CAUSED AND ON ANY THEORY OF LIABILITY, WHETHER IN CONTRACT, STRICT LIABILITY, OR TORT (INCLUDING NEGLIGENCE OR OTHERWISE) ARISING IN ANY WAY OUT OF THE USE OF THIS SOFTWARE, EVEN IF ADVISED OF THE POSSIBILITY OF SUCH DAMAGE."
  n1 = global read "AlliGator Globals.vi" "Alligator version"() -> (w9:string)
  n2 = case shown="\"GUI:Set Verbose Settings Mode\"" "AlliGator Q Event in" {
    tunnel: [_ _ _ _ _ _ _ _ _ _ _ _ TRUE _ _ _ _ _ _ _ _ _ _ _ _ _ _ _ _ _] -> w10
    tunnel: "Data" -> [_ _ _ _ w114 w122 w128 _ _ _ w166 w193 _ w232 _ w247 w258 w286 w291 w299 _ _ w340 w360 w366 w386 w392 w400 w412 w421]
    tunnel: "AlliGator Q Elements in" -> [w23 w42 w73 w102 w110 w124 w131 w135 w146 w155 w171 w195 _ w234 w241 w249 w261 w288 w295 w302 w310 w322 w339 w359 w371 w384 w396 w406 w415 w424]
    tunnel: [w23 w42 w73 w102 w111 w124 w131 w135 w146 w154 w171 w194 T6[] [] ("Named Q Element") w234 w241 w249 w261 w288 w295 w302 w310 w322 w338 w359 w370 w383 w396 w406 w415 w424] -> w12
    tunnel: "VI in" -> [_ w46 w59 _ _ w120 w126 _ _ w153 _ w188 w222 _ _ _ _ _ w289 w297 w303 _ _ _ _ _ _ _ _ _]
    tunnel: w9 -> [_ _ _ _ _ _ _ _ _ _ _ _ w221 _ _ _ _ _ _ _ _ _ _ _ _ _ _ _ _ _]
    tunnel: [w22 w45 w57 w100 w117 w119 w125 w134 w145 w156 w170 w182 w220 w233 w240 w248 w260 w287 w294 w296 w305 w321 w332 w355 w363 w387 w395 w405 w414 w423] -> w8
    tunnel: "Script" -> [w22 _ w56 w100 w117 w119 w125 w134 w145 w156 w170 w172 w220 w233 w240 w248 w260 w287 w294 w296 _ w321 w332 w355 w363 w387 w395 w405 w414 w423]
    tunnel: "error in (no error)" -> [w21 _ w55 w99 _ w118 w130 w133 w144 w152 w158 _ _ w227 w239 _ w257 _ w293 w301 w309 w320 _ w354 _ _ w394 w404 w409 w418]
    tunnel: [w21 w36 w71 w99 w109 w118 w130 w133 w144 w151 w157 w183 w211 w228 w239 w243 w254 w277 w293 w301 w304 w320 w331 w354 w362 w377 w394 w404 w410 w419] -> w1
    tunnel: "AlliGator Ctrl Refnums" -> [_ w30 w66 w98 _ _ _ _ _ w148 _ w187 w206 _ _ _ w253 w283 _ _ _ _ _ w353 _ w376 _ _ _ _]
    tunnel: "AlliGator IV DVR" -> [w20 w27 w63 w95 w108 w123 w129 w132 w143 w150 w169 w180 w205 w230 w238 w242 w259 w276 w292 w300 w308 w319 w328 w349 w361 w374 w393 w403 w413 w422]
    tunnel: [w20 w27 w63 w90 w106 w123 w129 w132 w141 w149 w169 w179 w205 w229 w237 w242 w259 w276 w292 w300 w307 w317 w327 w345 w361 w375 w393 w403 w413 w422] -> w19
    tunnel: [_ w25 w62 _ _ _ _ _ _ w147 _ _ w204 w226 _ _ _ _ _ _ _ _ _ _ _ _ _ _ _ _] -> w6
    frame "---- GUI ----", Default {
      # "\"---- GUI ----\""
    }
    frame "GUI:Abort" {
      w45 = FALSE  # Script
      w41 = TRUE ("Get(F)/Set")
      w38 = FALSE ("Visible")
      # "\"Abort\""
      n3 = Unbundle By Name(w30) -> ("Other AlliGator Ctrl Refnums.CPU"=w29:refnum<vi>)
      n4 = call "AlliGator Settings Storage.vi"("AlliGator Settings List"=AlliGator_Settings_List."Miscellaneous:Beep after Script") -> ("Error Out"=w47:errorcluster, "Variant Data out"=w49:variant)  [unwired: 9 in]
      n5 = global write "AlliGator Abort.vi" "Abort?"(w38) -> ()
      n6 = call-poly "Variant to Data.vi"("Variant"=w49) -> ("Value"=w48:bool)  [unwired: 8 in]
      n7 = call "Hide Animated Busy Icon with Message and Abort Button.vi"("Message"="Script aborted...", "Target VI reference"=w46, "Error In"=w47) -> ("Error Out"=w31:errorcluster)  [unwired: 16 in]
      n8 = call "Alligator Variables Storage.vi"("Get(F)/Set"=w41, "AlliGator Variable"=AlliGator_Variables_List."GUI:Script in progress" ("Alligator Variable"), "Data in"=w38) -> ("Error Out"=w33:errorcluster)  [unwired: 6 in, 2 out]
      n9 = call "Alligator Variables Storage.vi"("Get(F)/Set"=w41, "AlliGator Variable"=AlliGator_Variables_List."GUI:Playback" ("Alligator Variable"), "Data in"=w38) -> ("Error Out"=w34:errorcluster)  [unwired: 6 in, 2 out]
      n10 = call "Alligator Variables Storage.vi"("Get(F)/Set"=w41, "AlliGator Variable"=AlliGator_Variables_List."GUI:Loop Playback" ("Alligator Variable"), "Data in"=w38) -> ("Error Out"=w35:errorcluster)  [unwired: 6 in, 2 out]
      n11 = call "Current Date & Time String (High Precision).vi"() -> ("Error Out"=w37:errorcluster, "time string"=w43:string, "date string"=w44:string)  [unwired: 8 in, 1 out]
      n12 = case shown="True" w48 {
        frame False {
        }
        frame True {
          n13 = call "Play Abort Sound.vi"() -> ()  [unwired: 27 in, 1 out]
        }
      }
      n14 = property class="DigNum (strict)"(reference=w29, "Visible"=FALSE) -> ()  [unwired: 1 in, 2 out]
      n15 = call "Alligator Variables Storage.vi"("Get(F)/Set"=w41, "AlliGator Variable"=AlliGator_Variables_List."Destination File Path" ("Alligator Variable"), "Error In"=w33, "Data in"=path "") -> ("Error Out"=w32:errorcluster)  [unwired: 5 in, 2 out]
      n16 = Format Into String(format string="Operation aborted by user on %s at %s", error in=w37, w44, w43) -> (resulting string=w25:string, error out=w24:errorcluster)  [unwired: 1 in]
      n17 = Merge Errors(w31, w32, w34, w35, w24) -> (w36:errorcluster)
    }
    frame "GUI:End Script" {
      w57 = FALSE  # Script
      w79 = TRUE ("Get(F)/Set")
      w64 = FALSE ("Visible")
      # "\"End Script\""
      n18 = call "AlliGator Settings Storage.vi"("AlliGator Settings List"=AlliGator_Settings_List."Miscellaneous:Beep after Script", "Error In"=w55) -> ("Error Out"=w74:errorcluster, "Variant Data out"=w76:variant)  [unwired: 8 in]
      n19 = Unbundle By Name(w66) -> ("Other AlliGator Ctrl Refnums.CPU"=w65:refnum<vi>)
      n20 = call-poly "Variant to Data.vi"("Variant"=w76) -> ("Value"=w75:bool)  [unwired: 8 in]
      n21 = call "Hide Animated Busy Icon with Message and Abort Button.vi"("Target VI reference"=w59, "Error In"=w74, "Abort Button Name (Abort)"="Abort") -> ("Error Out"=w72:errorcluster)  [unwired: 16 in]
      n22 = call "Alligator Variables Storage.vi"("Get(F)/Set"=w79, "AlliGator Variable"=AlliGator_Variables_List."GUI:Script in progress" ("Alligator Variable"), "Data in"=w64) -> ("Error Out"=w70:errorcluster)  [unwired: 6 in, 2 out]
      n23 = call "Alligator Variables Storage.vi"("Get(F)/Set"=w79, "AlliGator Variable"=AlliGator_Variables_List."GUI:Loop Playback" ("Alligator Variable"), "Data in"=w64) -> ("Error Out"=w68:errorcluster)  [unwired: 6 in, 2 out]
      n24 = call "Alligator Variables Storage.vi"("Get(F)/Set"=w79, "AlliGator Variable"=AlliGator_Variables_List."GUI:Playback" ("Alligator Variable"), "Data in"=w64) -> ("Error Out"=w69:errorcluster)  [unwired: 6 in, 2 out]
      n25 = call "Hide Animated Busy Icon with Message and Abort Button.vi"("Target VI reference"=w59, "Error In"=w72, "Abort Button Name (Abort)"="Abort Fit") -> ("Error Out"=w60:errorcluster)  [unwired: 16 in]
      n26 = case shown="True" w75 {
        frame False {
        }
        frame True {
          n27 = call "Play End of Task Sound.vi"() -> ()  [unwired: 27 in, 1 out]
        }
      }
      n28 = case shown="False" w56 {
        tunnel: [_ w83] -> w67
        tunnel: [_ w82] -> w62
        frame False {
        }
        frame True {
          n29 = call "Current Date & Time String (High Precision).vi"() -> ("Error Out"=w84:errorcluster, "time string"=w85:string, "date string"=w86:string)  [unwired: 8 in, 1 out]
          n30 = Format Into String(format string="Script stopped on %s at %s", error in=w84, w86, w85) -> (resulting string=w82:string, error out=w83:errorcluster)  [unwired: 1 in]
        }
      }
      n31 = property class="DigNum (strict)"(reference=w65, "Visible"=w64) -> ()  [unwired: 1 in, 2 out]
      n32 = global write "Abort Fit Global.vi" "Abort Fit"(w57) -> ()
      n33 = global write "AlliGator Abort.vi" "Abort?"(w57) -> ()
      n34 = Merge Errors(w60, w70, w69, w68, w67) -> (w71:errorcluster)
    }
    frame "GUI:End Timing" {
      # "\"End Timing\""
      n35 = Unbundle By Name(w98) -> ("Other AlliGator Ctrl Refnums.CPU"=w97:refnum<vi>)
      n36 = call "AlliGator IV Start Time.vi"("Get (F)/ Set (T)"=FALSE, "AlliGator IV DVR in"=w95) -> ("error out"=w91:errorcluster, "Start Time"=w94:dbl, "AlliGator IV DVR out"=w92:refnum<data-value>)  [unwired: 7 in]
      n37 = call <vilib>:"High Resolution Relative Seconds.vi"() -> ("relative seconds"=w93:dbl)
      n38 = Subtract(x=w93, y=w94) -> (x-y=w101:dbl)
      n39 = node(w101) -> (w96:dbl[unit])
      n40 = call "AlliGator IV Start Time.vi"("Get (F)/ Set (T)"=TRUE, "error in (no error)"=w91, "Start Time"=w93, "AlliGator IV DVR in"=w92) -> ("AlliGator IV DVR out"=w90:refnum<data-value>)  [unwired: 5 in, 2 out]
      n41 = property class="DigNum (strict)"(reference=w97, "Value"=w96) -> ()  [unwired: 1 in, 2 out]
    }
    frame "GUI:Gate Image Slide Changed" {
      # "\"Time Gate Slider Changed\""
      n42 = call-poly "Variant to Data.vi"("Variant"=w114) -> ("U16 Value"=w104:u16)  [unwired: 8 in]
      n43 = call "Alligator Variables Storage.vi"("Get(F)/Set"=TRUE, "AlliGator Variable"=AlliGator_Variables_List."X_Time Gate Slider" ("Alligator Variable"), "Data in"=w104) -> ("Error Out"=w107:errorcluster)  [unwired: 6 in, 2 out]
      n44 = call "AlliGator IV Gate Image Slide.vi"("Get (F)/ Set (T)"=TRUE, "error in (no error)"=w107, "Gate Image Slide"=w104, "AlliGator IV DVR in"=w108) -> ("error out"=w105:errorcluster, "AlliGator IV DVR out"=w106:refnum<data-value>)  [unwired: 5 in, 1 out]
      n45 = call-poly "AlliGator Add Action(s) to Stack.vi"("Elements Order in Action Stack (Default: 2 BEFORE 1)"=Alligator_Elements_Order_in_Action_Stack."Enqueue 2 AFTER 1", "Error In"=w105, "Alligator Atomic Action"=T6 {"AlliGator Q Event"=enum."Image:Update Image Profile Plots", "Data"=variant}, "Alligator Queue Element 1"=w110) -> ("Error Out"=w109:errorcluster, "Alligator Queue Element 1 (+ 2)"=w111:T6[])  [unwired: 6 in]
    }
    frame "GUI:Hide Busy Icon & Abort Button" {
      # "\"GUI:Hide Busy Icon & Abort Button\""
      n46 = call-poly "Variant to Data.vi"("Variant"=w122) -> ("String"=w121:string)  [unwired: 8 in]
      n47 = call "Hide Animated Busy Icon with Message and Abort Button.vi"("Already active? (F)"=w119, "Message"=w121, "Target VI reference"=w120) -> ()  [unwired: 16 in, 1 out]
    }
    frame "GUI:Hide Busy Icon" {
      # "\"GUI:Hide Busy Icon\""
      n48 = call-poly "Variant to Data.vi"("Variant"=w128) -> ("String"=w127:string)  [unwired: 8 in]
      n49 = call "Hide Animated Busy Icon with Message.vi"("Already active? (F)"=w125, "Message"=w127, "Target VI reference"=w126) -> ()  [unwired: 8 in, 1 out]
    }
    frame "GUI:Idle" {
      # "\"Idle\""
    }
    frame "GUI:Increment Dataset Index" {
      # "Increment Dataset Index"
      n50 = call "AlliGator IV Current Dataset.vi"("Get (F)/ Set (T)"=FALSE, "AlliGator IV DVR in"=w143) -> ("error out"=w138:errorcluster, "Current Dataset"=w140:i32, "AlliGator IV DVR out"=w142:refnum<data-value>)  [unwired: 7 in]
      n51 = Increment(x=w140) -> (x+1=w139:i32)
      n52 = call "AlliGator IV Current Dataset.vi"("Get (F)/ Set (T)"=TRUE, "error in (no error)"=w138, "Current Dataset"=w139, "AlliGator IV DVR in"=w142) -> ("AlliGator IV DVR out"=w141:refnum<data-value>)  [unwired: 5 in, 2 out]
    }
    frame "GUI:Initialization" {
      # "\"Initialization\""
      n53 = call "AlliGator GUI Initialization.vi"("VI in"=w153, "error in (no error)"=w152, "AlliGator Ctrl Refnums"=w148, "AlliGator IV DVR"=w150, "AlliGator Q Elements in"=w155) -> ("error out"=w151:errorcluster, "Message"=w147:string, "AlliGator IV DVR"=w149:refnum<data-value>, "AlliGator Q Elements out"=w154:T6[])  [unwired: 3 in]
    }
    frame "GUI:Open Window" {
      # "\"GUI:Open Window\""
      n54 = Variant To Data(error in=w158, type=T21 {"AlliGator Windows"=enum."AlliGator Window", "Open Window Options"={"Bring To Front (T)"=FALSE, "Start Hidden? (F)"=FALSE, "Activate? (T)"=FALSE}} ("output cluster"), Variant=w166) -> (data=w164:T21, error out=w162:errorcluster)
      n55 = Unbundle By Name(w164) -> ("AlliGator Windows"=w163:T22, "Open Window Options.Bring To Front (T)"=w161:bool, "Open Window Options.Start Hidden? (F)"=w160:bool, "Open Window Options.Activate? (T)"=w159:bool)
      n56 = call "AlliGator Get Ancillary Window Path.vi"("Error In"=w162, "AlliGator Window"=w163) -> ("Error Out"=w167:errorcluster, "VI Path"=w168:path)  [unwired: 8 in]
      n57 = call "Run Vi.vi"("Bring To Front (T)"=w161, "VI Path"=w168, "error in (no error)"=w167, "Start Hidden? (F)"=w160, "Activate? (T)"=w159) -> ("error out"=w157:errorcluster)  [unwired: 3 in, 1 out]
    }
    frame "GUI:Playback Script" {
      w182 = TRUE ("Visible")
      # "\"Playback Script\""
      n58 = Unbundle By Name(w187) -> ("Phasor Plot Ctrl Refnums.Save Phasor Plot"=w190:refnum<vi>, "Dataset Control Refnums.Save Image"=w186:refnum<vi>)
      n59 = call-poly "Variant to Data.vi"("Variant"=w193) -> ("Value"=w192:bool)  [unwired: 8 in]
      n60 = Unbundle By Name(w187) -> ("Dataset Control Refnums.Displayed Image"=w174:refnum<vi>, "Other AlliGator Ctrl Refnums.CPU"=w181:refnum<vi>, "Dataset Control Refnums.Time Point Slide"=w175:refnum<vi>)
      n61 = property class="Bool (strict)"(reference=w186) -> ("Value"=w185:bool)  [unwired: 1 in, 2 out]
      n62 = call "AlliGator IV Dataset Series Folder & Type.vi"("Get (F)/ Set (T)"=FALSE, "AlliGator IV DVR in"=w180) -> ("AlliGator Data Series Type"=w178:T30, "AlliGator IV DVR out"=w179:refnum<data-value>, "[Time-Series Path]"=w177:path[])  [unwired: 5 in, 2 out]
      n63 = property class="Enum (strict)"(reference=w174) -> ("Value"=w173:T31)  [unwired: 1 in, 2 out]
      n64 = property class="Bool (strict)"(reference=w190) -> ("Value"=w189:bool)  [unwired: 1 in, 2 out]
      n65 = call "AlliGator Playback Time-Gated Data Series v2.vi"("Alligator Queue Elements in"=w195, "Save Image with Overlay"=w185, "Save Phasor Plot with Overlay"=w189, "Series Paths"=w177, "Type of Displayed Image"=w173, "Time Slider Refnum"=w175, "AlliGator Data Series Type"=w178, "Playback (F)/Loop (T)"=w192) -> ("Alligator Queue Elements out"=w194:T6[], "Error Out"=w191:errorcluster)  [unwired: 6 in]
      n66 = call "Show Animated Busy Icon with Message and Abort Button.vi"("Already active? (F)"=w172, "Target VI reference"=w188, "Error In"=w191) -> ("Error Out"=w184:errorcluster)  [unwired: 16 in]
      n67 = property class="DigNum (strict)"(reference=w181, error in=w184, "Visible"=w182) -> (error out=w183:errorcluster)  [unwired: 1 out]
    }
    frame "GUI:Quit" {
      # "\"Quit\""
      n68 = call "Formula Aliases Storage.vi"() -> ("Descriptions Array"=w199:string[], "Definitions Array"=w200:string[], "Aliases Array"=w201:string[])  [unwired: 8 in, 1 out]
      n69 = call "Open-Save Alias Definitions.vi"("Open (F)/ Save"=TRUE, "Descriptions Array in"=w199, "Definitions Array in"=w200, "Aliases Array in"=w201) -> ("Error Out"=w197:errorcluster)  [unwired: 3 in, 4 out]
      n70 = call "AlliGator Quit Source Image ROI Manager.vi"() -> ("Error Out"=w214:errorcluster)  [unwired: 11 in]
      n71 = call "AlliGator Quit Phasor Plot Image ROI Manager.vi"() -> ("Error Out"=w215:errorcluster)  [unwired: 11 in]
      n72 = call "AlliGator Save-Load Settings.vi"("Load(F)/Save (T)"=TRUE, "Error In"=w197, "AlliGator Refnum in"=w222) -> ("Error Out"=w213:errorcluster)  [unwired: 7 in, 1 out]
      n73 = call "AlliGator Hide Path Drop Boxes.vi"("Hide (F)/Show"=FALSE, "AlliGator Ctrl Refnums"=w206) -> ()  [unwired: 9 in, 1 out]
      n74 = Merge Errors(w213, w214, w215) -> (w212:errorcluster)
      n75 = call "Delete Notebook Backup on Quit.vi"("Main VI Name"="AlliGator" ("Sender")) -> ("Error Out"=w217:errorcluster)  [unwired: 10 in]
      n76 = call "AlliGator Clear Variables.vi"("Error In"=w212) -> ("Error Out"=w210:errorcluster, "Message"=w203:string)  [unwired: 9 in]
      n77 = call "Current Date & Time String (High Precision).vi"() -> ("time string"=w218:string, "date string"=w219:string)  [unwired: 8 in, 2 out]
      n78 = call "Embedded Progress Bar Q.vi"("Progress Bar Queue Name"="AlliGator Progress Bar Q") -> ("Progress Bar Queue"=w208:refnum<queue>)  [unwired: 6 in]
      n79 = Format Into String(format string="\nAlliGator %s stopped on %s at %s" ("initial string"), initial string=w203, w221, w219, w218) -> (resulting string=w204:string)  [unwired: 1 in, 1 out]
      n80 = Enqueue Element(queue=w208, element=T24 {"Action"="Quit", "Value"=0.0} ("Progress Bar Q Element")) -> ()  [unwired: 2 in, 3 out]
      n81 = Merge Errors(w210, w217) -> (w211:errorcluster)
    }
    frame "GUI:Send Parameters JSON Strings to Clipboard" {
      # "\"GUI:Send Parameters JSON Strings to Clipboard\""
      n82 = call-poly "Variant to Data.vi"("Variant"=w232) -> ("Value"=w231:bool)  [unwired: 8 in]
      n83 = call "AlliGator Export Plugin Parameters to Clipboard.vi"("Error In"=w227, "Parameter Names only"=w231, "AlliGator IV DVR"=w230) -> ("Error Out"=w228:errorcluster, "Message"=w226:string, "AlliGator IV DVR"=w229:refnum<data-value>)  [unwired: 6 in]
    }
    frame "GUI:Set Dataset Index to -1" {
      # "\"Set Dataset Index to -1\""
      n84 = call "AlliGator IV Current Dataset.vi"("Get (F)/ Set (T)"=TRUE, "Current Dataset"=-1, "AlliGator IV DVR in"=w238) -> ("AlliGator IV DVR out"=w237:refnum<data-value>)  [unwired: 6 in, 2 out]
    }
    frame "GUI:Set Gate Step" {
      # "#todo: This does not update the Settings Window"
      # "\"Set Gate Step\""
      n85 = call-poly "Variant to Data.vi"("Variant"=w247) -> ("Value"=w246:i32)  [unwired: 8 in]
      n86 = call "AlliGator Settings Storage.vi"("Get(F)/Set"=TRUE, "AlliGator Settings List"=AlliGator_Settings_List."Data Information:Gate Step", "Variant Data in"=w246) -> ("Error Out"=w243:errorcluster)  [unwired: 7 in, 1 out]
    }
    frame "GUI:Set Phasor Frequency" {
      # "\"GUI:Set Phasor Frequency\""
      n87 = Variant To Data(error in=w257, type=dbl[unit] 0.0 ("Phasor Frequency"), Variant=w258) -> (data=w252:dbl[unit], error out=w255:errorcluster)
      n88 = call "AlliGator Phasor Frequency.vi"() -> ("Phasor Frequency"=w251:dbl[unit])
      n89 = Not Equal?(x=w252, y=w251) -> (x != y?=w250:bool)
      n90 = case shown="True" w250 {
        tunnel: w255 -> [w262 w272]
        tunnel: [w262 w271] -> w254
        tunnel: w253 -> [_ w269]
        tunnel: w252 -> [_ w263]
        frame False {
        }
        frame True {
          w273 = TRUE ("ON/OFF")
          w265 = "Program" ("Sender")
          n91 = call "AlliGator Update Settings & Control.vi"("Control Label"="Phasor Graph Frequency", "Error In"=w272, "Value"=w263, "Sender"=w265) -> ("Error Out"=w267:errorcluster)  [unwired: 7 in]
          n92 = Unbundle By Name(w269) -> ("Other AlliGator Ctrl Refnums.State Indicators"=w268:refnum<vi>)
          n93 = call "AlliGator Update Settings & Control.vi"("Control Label"="Phasor Plot Frequency", "Error In"=w267, "Value"=w263, "Sender"=w265) -> ("Error Out"=w266:errorcluster)  [unwired: 7 in]
          n94 = call "AlliGator Get-Set State Indicators.vi"("State Indicators Refnum"=w268, "AlliGator State Indicators List"=AlliGator_State_Indicators_List."Phasor Plot Update Needed", "Error In"=w266, "ON/OFF"=w273, "Set (T)/Get"=w273) -> ("Error Out"=w271:errorcluster)  [unwired: 8 in, 2 out]
        }
      }
    }
    frame "GUI:Set State Indicator" {
      # "\"Set State Indicator\""
      n95 = Variant To Data(type=T26 {"State Indicators List"=enum."Phasor Calibration Defined", "ON/OFF"=FALSE, "# Defined IRFs"=0} ("Cluster"), Variant=w286) -> (data=w284:T26, error out=w279:errorcluster)  [unwired: 1 in]
      n96 = Unbundle By Name(w284) -> ("# Defined IRFs"=w278:i32, "State Indicators List"=w281:T25, "ON/OFF"=w280:bool)
      n97 = Unbundle By Name(w283) -> ("Other AlliGator Ctrl Refnums.State Indicators"=w282:refnum<vi>)
      n98 = call "AlliGator Get-Set State Indicators.vi"("# Defined IRFs"=w278, "State Indicators Refnum"=w282, "AlliGator State Indicators List"=w281, "Error In"=w279, "ON/OFF"=w280, "Set (T)/Get"=TRUE) -> ("Error Out"=w277:errorcluster)  [unwired: 7 in, 2 out]
    }
    frame "GUI:Show Busy Icon & Abort Button" {
      # "\"GUI:Show Busy Icon & Abort Button\""
      n99 = call-poly "Variant to Data.vi"("Variant"=w291) -> ("String"=w290:string)  [unwired: 8 in]
      n100 = call "Show Animated Busy Icon with Message and Abort Button.vi"("Message"=w290, "Target VI reference"=w289) -> ()  [unwired: 17 in, 1 out]
    }
    frame "GUI:Show Busy Icon" {
      # "\"GUI:Show Busy Icon\""
      n101 = call-poly "Variant to Data.vi"("Variant"=w299) -> ("String"=w298:string)  [unwired: 8 in]
      n102 = call "Show Animated Busy Icon with Message.vi"("Already active? (F)"=w296, "Message"=w298, "Target VI Refnum"=w297) -> ()  [unwired: 8 in, 1 out]
    }
    frame "GUI:Start Script" {
      w305 = TRUE ("Get(F)/Set")
      # "This is the only place this is set and results in a failure to process decays\nloaded in the Decay Graph if no script has been run before"
      # "\"GUI:Start Script\""
      n103 = call "Show Animated Busy Icon with Message and Abort Button.vi"("Target VI reference"=w303, "Error In"=w309) -> ("Error Out"=w304:errorcluster)  [unwired: 17 in]
      n104 = disable-structure shown="Enabled" {
        disable-tunnel: w308 -> [w314 w315]
        disable-tunnel: [w313 w315] -> w307
        frame Disabled {
          n105 = call "AlliGator IV Valid Decay.vi"("Get (F)/ Set (T)"=TRUE, "Valid Decay"=TRUE, "AlliGator IV DVR in"=w314) -> ("AlliGator IV DVR out"=w313:refnum<data-value>)  [unwired: 6 in, 2 out]
        }
        frame Enabled {
        }
      }
      n106 = call "Alligator Variables Storage.vi"("Get(F)/Set"=w305, "AlliGator Variable"=AlliGator_Variables_List."GUI:Script in progress" ("Alligator Variable"), "Data in"=w305) -> ()  [unwired: 6 in, 3 out]
    }
    frame "GUI:Start Timing" {
      # "\"Start Timing\""
      n107 = call <vilib>:"High Resolution Relative Seconds.vi"() -> ("relative seconds"=w318:dbl)
      n108 = call "AlliGator IV Start Time.vi"("Get (F)/ Set (T)"=TRUE, "Start Time"=w318, "AlliGator IV DVR in"=w319) -> ("AlliGator IV DVR out"=w317:refnum<data-value>)  [unwired: 6 in, 2 out]
    }
    frame "GUI:Time Series Slider Changed" {
      # "\"Time Series Slider Changed\""
      n109 = call-poly "Variant to Data.vi"("Variant"=w340) -> ("U16 Value"=w333:u16)  [unwired: 8 in]
      n110 = Decrement(x=w333) -> (x-1=w326:u16)
      n111 = call "AlliGator IV Dataset Series Folder & Type.vi"("Get (F)/ Set (T)"=FALSE, "AlliGator IV DVR in"=w328) -> ("error out"=w325:errorcluster, "[Time-Series Path]"=w330:path[])  [unwired: 5 in, 3 out]
      n112 = Index Array(array=w330, index=w326) -> (element=w335:path)
      n113 = call "AlliGator IV Current Dataset.vi"("Get (F)/ Set (T)"=TRUE, "error in (no error)"=w325, "Current Dataset"=w326, "AlliGator IV DVR in"=w328) -> ("error out"=w323:errorcluster, "AlliGator IV DVR out"=w327:refnum<data-value>)  [unwired: 5 in, 1 out]
      n114 = Bundle By Name(cluster=T6 {"AlliGator Q Event"=enum."Files:New Folder Selected", "Data"=variant} ("Alligator Atomic Action"), "Data"=w335) -> (w336:T6)
      n115 = call-poly "AlliGator Add Action(s) to Stack.vi"("Elements Order in Action Stack (Default: 2 BEFORE 1)"=Alligator_Elements_Order_in_Action_Stack."Enqueue 2 BEFORE 1", "Error In"=w323, "Alligator Atomic Action"=w336, "Alligator Queue Element 1"=w339) -> ("Error Out"=w331:errorcluster, "Alligator Queue Element 1 (+ 2)"=w338:T6[])  [unwired: 6 in]
    }
    frame "GUI:Time Series Slider Moved" {
      w344 = FALSE ("Get (F)/ Set (T)")
      # "we are only updating the folder name\nuntil the user releases the slider"
      # "\"Time Series Slider Moved\""
      n116 = Unbundle By Name(w353) -> ("Dataset Control Refnums.Current Time Stamp"=w351:refnum<vi>, "Dataset Control Refnums.Current Data"=w341:refnum<vi>)
      n117 = call "AlliGator IV Time Series Timestamps & Current Dataset.vi"("Get (F)/ Set"=w344, "AlliGator IV DVR in"=w349) -> ("error out"=w343:errorcluster, "[Time-Series Timestamps]"=w348:dbl[], "AlliGator IV DVR out"=w346:refnum<data-value>)  [unwired: 6 in, 1 out]
      n118 = call-poly "Variant to Data.vi"("Variant"=w360) -> ("U16 Value"=w356:u16)  [unwired: 8 in]
      n119 = Decrement(x=w356) -> (x-1=w357:u16)
      n120 = call "AlliGator IV Dataset Series Folder & Type.vi"("Get (F)/ Set (T)"=w344, "error in (no error)"=w343, "AlliGator IV DVR in"=w346) -> ("error out"=w342:errorcluster, "AlliGator IV DVR out"=w345:refnum<data-value>, "[Time-Series Path]"=w347:path[])  [unwired: 4 in, 2 out]
      n121 = Index Array(array=w348, index=w357) -> (element=w350:dbl)
      n122 = Index Array(array=w347, index=w357) -> (element=w358:path)
      n123 = Strip Path(path=w358) -> (name=w352:string)  [unwired: 1 out]
      n124 = property class="DigNum (strict)"(reference=w351, error in=w342, "Value"=w350) -> ()  [unwired: 2 out]
      n125 = property class="Str"(reference=w341, error in=w342, "Value"=w352) -> ()  [unwired: 2 out]
    }
    frame "GUI:Toggle Playback or Loop" {
      # "\"Toggle Playback or Loop\""
      n126 = call-poly "Variant to Data.vi"("Variant"=w366) -> ("Value"=w365:bool)  [unwired: 8 in]
      n127 = call "AlliGator Toggle (Loop) Playback.vi"("Playback (F)/Loop (T)"=w365) -> ("Error Out"=w367:errorcluster)  [unwired: 8 in]
      n128 = Bundle By Name(cluster=T6 {"AlliGator Q Event"=enum."GUI:Playback Script", "Data"=variant} ("Alligator Atomic Action"), "Data"=w365) -> (w368:T6)
      n129 = call "AlliGator Add Single Action to Stack.vi"("Elements Order in Action Stack (Default: 2 BEFORE 1)"=Alligator_Elements_Order_in_Action_Stack."Enqueue 2 BEFORE 1", "Error In"=w367, "Alligator Atomic Action"=w368, "Alligator Queue Element 1"=w371) -> ("Error Out"=w362:errorcluster, "Alligator Queue Element 1 (+ 2)"=w370:T6[])  [unwired: 6 in]
    }
    frame "GUI:Type of Displayed Image Changed" {
      # "\"Type of Displayed Image Changed\""
      n130 = Unbundle By Name(w376) -> ("Dataset Control Refnums.Displayed Image"=w372:refnum<vi>, "Dataset Control Refnums.Gate Image Slide"=w379:refnum<vi>)
      n131 = Variant To Data(type=AlliGator_Displayed_Image."Single Gate" ("NewVal"), Variant=w386) -> (data=w378:T27, error out=w380:errorcluster)  [unwired: 1 in]
      n132 = call "AlliGator Update Gate Image Slide.vi"("Displayed Image"=w372, "error in (no error)"=w380, "Type of Image"=w378, "Gate Image Slide refnum"=w379, "AlliGator IV DVR in"=w374) -> ("error out"=w373:errorcluster, "AlliGator IV DVR out"=w375:refnum<data-value>)  [unwired: 5 in]
      n133 = call-poly "AlliGator Add Action(s) to Stack.vi"("Elements Order in Action Stack (Default: 2 BEFORE 1)"=Alligator_Elements_Order_in_Action_Stack."Enqueue 2 BEFORE 1", "Error In"=w373, "Alligator Atomic Action"=T6 {"AlliGator Q Event"=enum."Image:Update Image Profile Plots", "Data"=variant}, "Alligator Queue Element 1"=w384) -> ("Error Out"=w377:errorcluster, "Alligator Queue Element 1 (+ 2)"=w383:T6[])  [unwired: 6 in]
    }
    frame "GUI:Start Test Script" {
      # "GUI:Start Test Script"
      n134 = call-poly "Variant to Data.vi"("Variant"=w392) -> ("String"=w391:string)  [unwired: 8 in]
      n135 = Bundle By Name(cluster=T29 {"Test String"="", "error"={"status"=FALSE, "code"=0, "source"=""}, "Status"=FALSE} ("output cluster"), "Test String"=w391) -> (w389:T29)
      n136 = call "AlliGator Test Internal Data.vi"("Test State"=T28."Store Test Name", "AlliGator Test Data"=w389) -> ()  [unwired: 8 in, 2 out]
    }
    frame "GUI:End Test Script" {
      # "\"GUI:End Test Script\""
      n137 = call-poly "Variant to Data.vi"("Variant"=w400) -> ("String"=w399:string)  [unwired: 8 in]
      n138 = Bundle By Name(cluster=T29 {"Test String"="", "error"={"status"=FALSE, "code"=0, "source"=""}, "Status"=FALSE} ("output cluster"), "Test String"=w399, "Status"=TRUE) -> (w401:T29)
      n139 = call "AlliGator Test Internal Data.vi"("Test State"=T28."Store Test Name", "AlliGator Test Data"=w401) -> ()  [unwired: 8 in, 2 out]
    }
    frame "GUI:Set Verbose Mode" {
      n140 = call-poly "Variant to Data.vi"("Variant"=w412) -> ("Value"=w411:bool)  [unwired: 8 in]
      n141 = call "AlliGator Settings Storage.vi"("Get(F)/Set"=TRUE, "AlliGator Settings List"=AlliGator_Settings_List."Miscellaneous:Verbose Mode", "Error In"=w409, "Variant Data in"=w411) -> ("Error Out"=w410:errorcluster)  [unwired: 6 in, 1 out]
    }
    frame "GUI:Set Verbose Settings Mode" {
      n142 = call-poly "Variant to Data.vi"("Variant"=w421) -> ("Value"=w420:bool)  [unwired: 8 in]
      n143 = call "AlliGator Settings Storage.vi"("Get(F)/Set"=TRUE, "AlliGator Settings List"=AlliGator_Settings_List."Miscellaneous:Verbose Settings Mode", "Error In"=w418, "Variant Data in"=w420) -> ("Error Out"=w419:errorcluster)  [unwired: 6 in, 1 out]
    }
  }
  "AlliGator IV DVR" <- w19
  "error out" <- w1
  "AlliGator Q Elements out" <- w12
  "Quit?" <- w10
  "Script?" <- w8
  n144 = call "Get Current Message Text Format.vi"("Text Format"=Text_Format_List."Message") -> ("Error Out"=w2:errorcluster, "Message Formatting"=w3:T2)  [unwired: 8 in]
  n145 = call "AlliGator Package Notebook Messages.vi"("Error In"=w2, "Message Formatting"=w3, "Message"=w6, "AlliGator Q Event in"="AlliGator Q Event in") -> ("[Notebook Message]"=→"[Notebook Message]":T1[])  [unwired: 6 in, 1 out]
